vi "STED Control V3.vi"() -> ()   [LabVIEW 2014]
uses:
  FPGA-7842R-Reference.ctl
  Scan Parameters.ctl
  Manual Controls V2.ctl
  <vilib>/Utility/miscctls.llb/LVRectTypeDef.ctl
  <vilib>/Utility/miscctls.llb/LVPositionTypeDef.ctl
  Laser Controls.ctl
  XY_Stage/StageStates.ctl
  Type Defs/Image Acquisition Parameters.ctl
  Detectors.ctl
  Stage Control.ctl
panel:
  in  "Manual Controls":T1={"Galvo 1 Position (I16)"=-280, "Galvo 2 Position (I16)"=0, "X Axis Voltage (I16)"=0, "Y Axis Voltage (I16)"=0, "Z Axis Voltage (I16)"=0, "Res Mirror Amp (I16)"=0, "Res Mirror Mute"=FALSE}
  in  "Stage Control":T2={"Halt"=FALSE, "Home"=FALSE, "Down Stage"=FALSE, "Right Stage"=FALSE, "Up Stage"=FALSE, "Left Stage"=FALSE, "Mode"=enum."Joystick", "X Position"=1.0, "Y Position"=1.0, "Step Size (um)"=enum."1", "Velocity"=enum."Low"} {"Y Position" min=1.0 max=24.0; "X Position" min=1.0 max=24.0}
  in  "Move XY Stage":bool
  in  "Autoscale Z":bool
  in  "Reset Zoom":bool
  in  "Zoom Out":bool
  in  "Zoom In":bool
  in  "Pan":bool
  in  "Remove Display":bool
  in  "Add Display":bool
  in  "Colormap 2":u16(ring) items=["Fire", "Gray", "Red", "Green", "Blue", "Cyan", "Magenta", "Yellow", "Red-White", "Green-White", "Blue-White", "Glow"]
  in  "Merge Tool":bool
  in  "Smooth Tool":bool
  out "Channel 6":sgl[][](graph)
  out "Channel 5":sgl[][](graph)
  out "Channel 4":sgl[][](graph)
  out "Channel 3":sgl[][](graph)
  out "Channel 2":sgl[][](graph)
  in  "Dual Screens":bool=TRUE
  in  "Detectors":T3
  in  "Laser Controls":T4 {"590 Power (V)" scale=0.0..3.0; "STED Power (V)" scale=0.0..5.0}
  in  "Save File Path":path
  in  "Capture":bool
  in  "show cursor":bool
  in  "Set Mode Offset":bool
  in  "Unused Axis Voltage":i16=16300
  out "Channel 1":sgl[][](graph)
  in  "Image Acquisition Parameters":T5={"Scan Type"=enum."Sample Scanning", "Scan Mode"=enum."XY", "Fast Axis Frequency (Hz)"=100.0, "Image Format"=128, "Line Accumulations"=1, "Frames Per Capture"=1, "Frames Accumulations"=1, "Image Dimension (um)"=[], "Number of Z Steps"=1, "Z Steps Size (um)"=1.0, "Pixel Size (nm)"=[]} {"Z Steps Size (um)" min=0.0; "Number of Z Steps" min=1; "Frames Accumulations" min=1; "Frames Per Capture" min=1; "Line Accumulations" min=1; "Image Format" items=["64 x 64"=64, "128 x 128"=128, "256 x 256"=256, "512 x 512"=512, "1024 x 1024"=1024, "2048 x 2048"=2048]}
  in  "Live":bool
  in  "Exit":bool
  # "XY"
  # "Z"
  # "Length"
  # "Height"
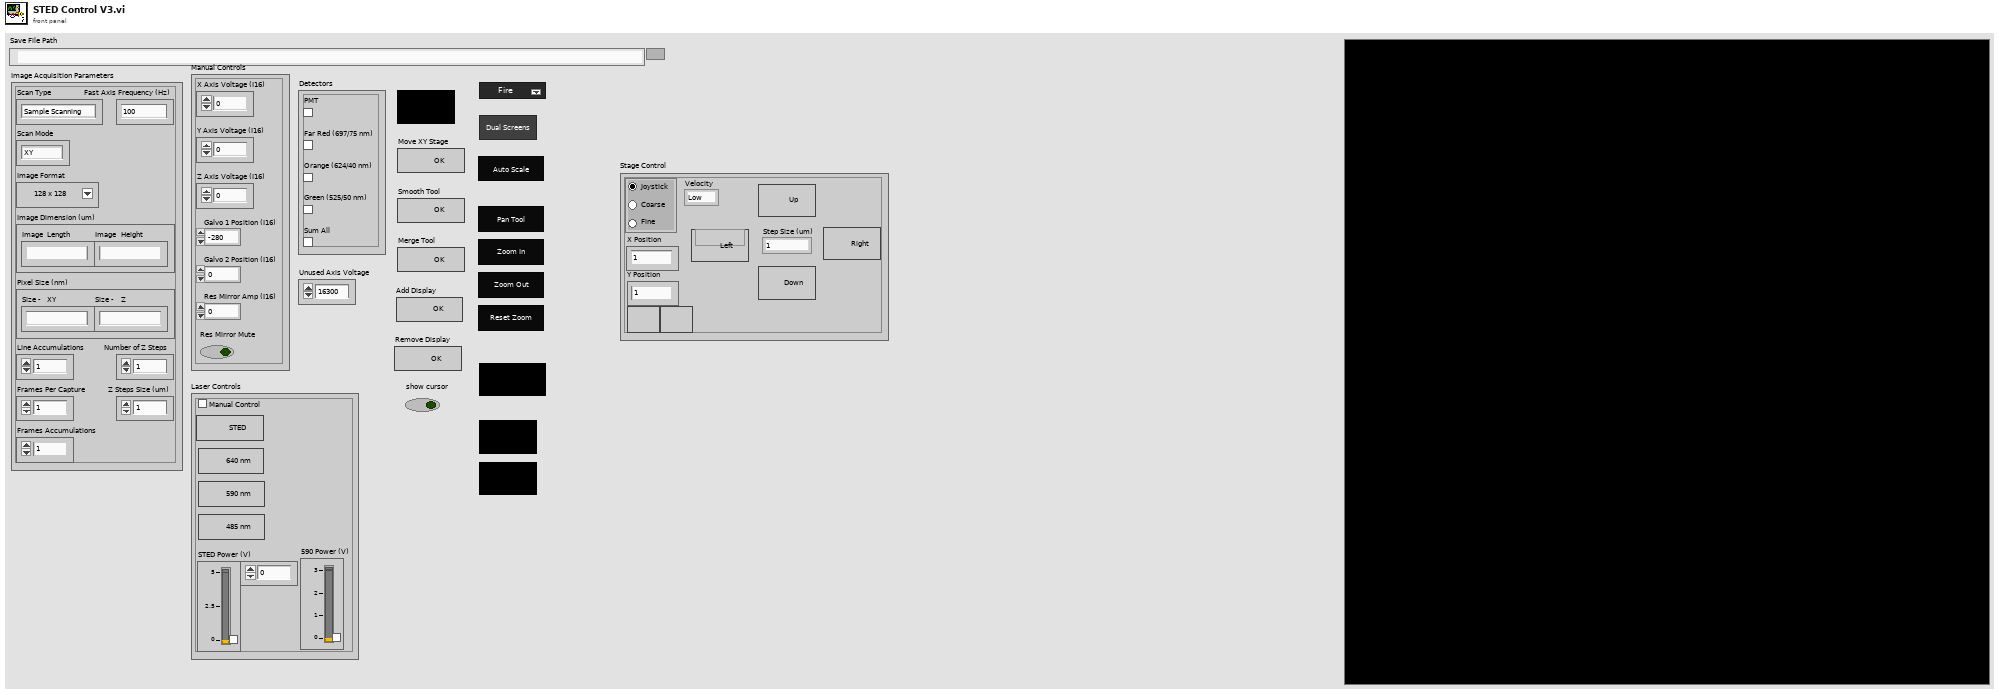
[diagram p1: front panel]
types:
  T1 = typedef "Manual Controls V2.ctl" = cluster{"Galvo 1 Position (I16)":i16, "Galvo 2 Position (I16)":i16, "X Axis Voltage (I16)":i16, "Y Axis Voltage (I16)":i16, "Z Axis Voltage (I16)":i16, "Res Mirror Amp (I16)":i16, "Res Mirror Mute":bool}
  T2 = typedef "Stage Control.ctl" = cluster{"Halt":bool, "Home":bool, "Down Stage":bool, "Right Stage":bool, "Up Stage":bool, "Left Stage":bool, "Mode":enum32{"Joystick", "Coarse", "Fine"}, "X Position":dbl, "Y Position":dbl, "Step Size (um)":enum16{"1", "2", "5", "10", "15", "20", "50", "100", "500"}, "Velocity":enum16{"Low", "Medium", "High"}}
  T3 = typedef "Detectors.ctl" = cluster{"PMT":bool, "Far Red (697/75 nm)":bool, "Orange (624/40 nm)":bool, "Green (525/50 nm)":bool, "Sum All":bool}
  T4 = typedef "Laser Controls.ctl" = cluster{"STED Power (V)":dbl, "590 Power (V)":dbl, "STED":bool, "640 nm":bool, "590 nm":bool, "485 nm":bool, "Manual Control":bool}
  T5 = typedef "Image Acquisition Parameters.ctl" = cluster{"Scan Type":enum16{"Sample Scanning", "Beam Scanning"}, "Scan Mode":enum16{"XY", "XZ", "YZ", "XYZ"}, "Fast Axis Frequency (Hz)":dbl, "Image Format":u16, "Line Accumulations":u16, "Frames Per Capture":u16, "Frames Accumulations":u16, "Image Dimension (um)":dbl[], "Number of Z Steps":u8, "Z Steps Size (um)":dbl, "Pixel Size (nm)":dbl[]}
  T6 = typedef "Scan Parameters.ctl" = cluster{"Fast_Ax_Amp_V":dbl, "Fast_Ax_Off_V":dbl, "Slow_Ax_Amp_V":dbl, "Slow_Ax_Off_V ":dbl, "Slow_Ax_Max_V_VperS":dbl, "Slow_Ax1_Del25ns":i32, "Slow_Ax2_Del25ns":i32, "Stage_X_Off_V":dbl, "Stage_Y_Off_V":dbl, "Stage_Z_Off_V":dbl, "Galvo1_Off_V":dbl, "Galvo2_Off_V":dbl, "Last_Scan_Mode":enum16{"XY", "XZ", "YZ", "XYZ"}, "Current_Scan_Mode":enum16{"XY", "XZ", "YZ", "XYZ"}, "Fly_Back_Lines":u16, "Linear_Ramp_End":u32, "Z_Step_I16":i16, "Z_Start_I16":i16, "Laser_States _U32":u32, "590_Voltage_I16":i16, "775_AOM_Volt_I16":i16, "Blanking OFF":bool, "Unused_Axis_I16":i16}
  T7 = typedef "FPGA-7842R-Reference.ctl" = enum16{"Stage Control", "Laser Control", "Unused Axis I16", "Exit", "Set Res Mirror", "Set Galvo", "Default", "Close FPGA", "Stop Waveforms", "Start Waveforms", "Initialize"}
  T8 = typedef "LVPositionTypeDef.ctl" = cluster{"Left":i32, "Top":i32}
  T9 = typedef "LVRectTypeDef.ctl" = cluster{"Left":i16, "Top":i16, "Right":i16, "Bottom":i16}
  T10 = enum32{"Invalid", "Standard", "Closed", "Hidden", "Minimized", "Maximized"}
  T11 = typedef "StageStates.ctl" = enum16{"POSITION", "MVR", "MOVE", "HALT", "ONTARGET", "ERROR", "EXIT", "HOME", "ZEROPOS", "NANOPOS", "QUIT", "SERVO", "JOYSTICK", "ANALOG"}
  T12 = typedef "LVRangeTypeDef.ctl" = cluster{"Minimum":dbl, "Maximum":dbl, "Increment":dbl, "Minor Increment":dbl, "Start":dbl}
  T13 = typedef "LVAllMonitorsDisplayTypeDef.ctl" = cluster{"Bounds":cluster{"Left":i16, "Top":i16, "Right":i16, "Bottom":i16}, "Depth":i16}[]
  T14 = cluster{"Bounds":cluster{"Left":i16, "Top":i16, "Right":i16, "Bottom":i16}, "Depth":i16}
  T15 = cluster{"Halt":bool, "Home":bool, "Down Stage":bool, "Right Stage":bool, "Up Stage":bool, "Left Stage":bool, "Mode":bool, "X Position":bool, "Y Position":bool, "Step Size (um)":bool, "Velocity":bool}
  T16 = enum16{"1", "2", "5", "10", "15", "20", "50", "100", "500"}
  T17 = typedef "Scanning Conversions.ctl" = cluster{"Stage X Axis (Volts/um)":dbl, "Stage Y Axis (Volts/um)":dbl, "Stage Z Axis (Volts/um)":dbl}
  T18 = typedef "IMAQ Image.ctl" = refnum<image>
  T19 = typedef "Waveform Data.ctl" = cluster{"Waveform Scan Parameters":cluster{"Scanning Mode":u8, "Fast Axis WF Length (Elements)":i32, "Fast Axis Sample Period (Ticks)":u32, "Slow Axis 1 WF Length (Elements)":i32, "Slow Axis 1 Sample Period (Ticks)":u32, "Slow Axis 1 Delay (25 ns) Steps":i32, "Slow Axis 2 WFLength (Elements)":i32, "Slow Axis 2 Sample Period (Ticks)":u32, "Slow Axis 2 Delay (25 ns) Steps":i32}, "Fast Axis Waveform":dbl[], "Slow Axis 1 Waveform":dbl[], "Slow Axis 2 Waveform":dbl[]}
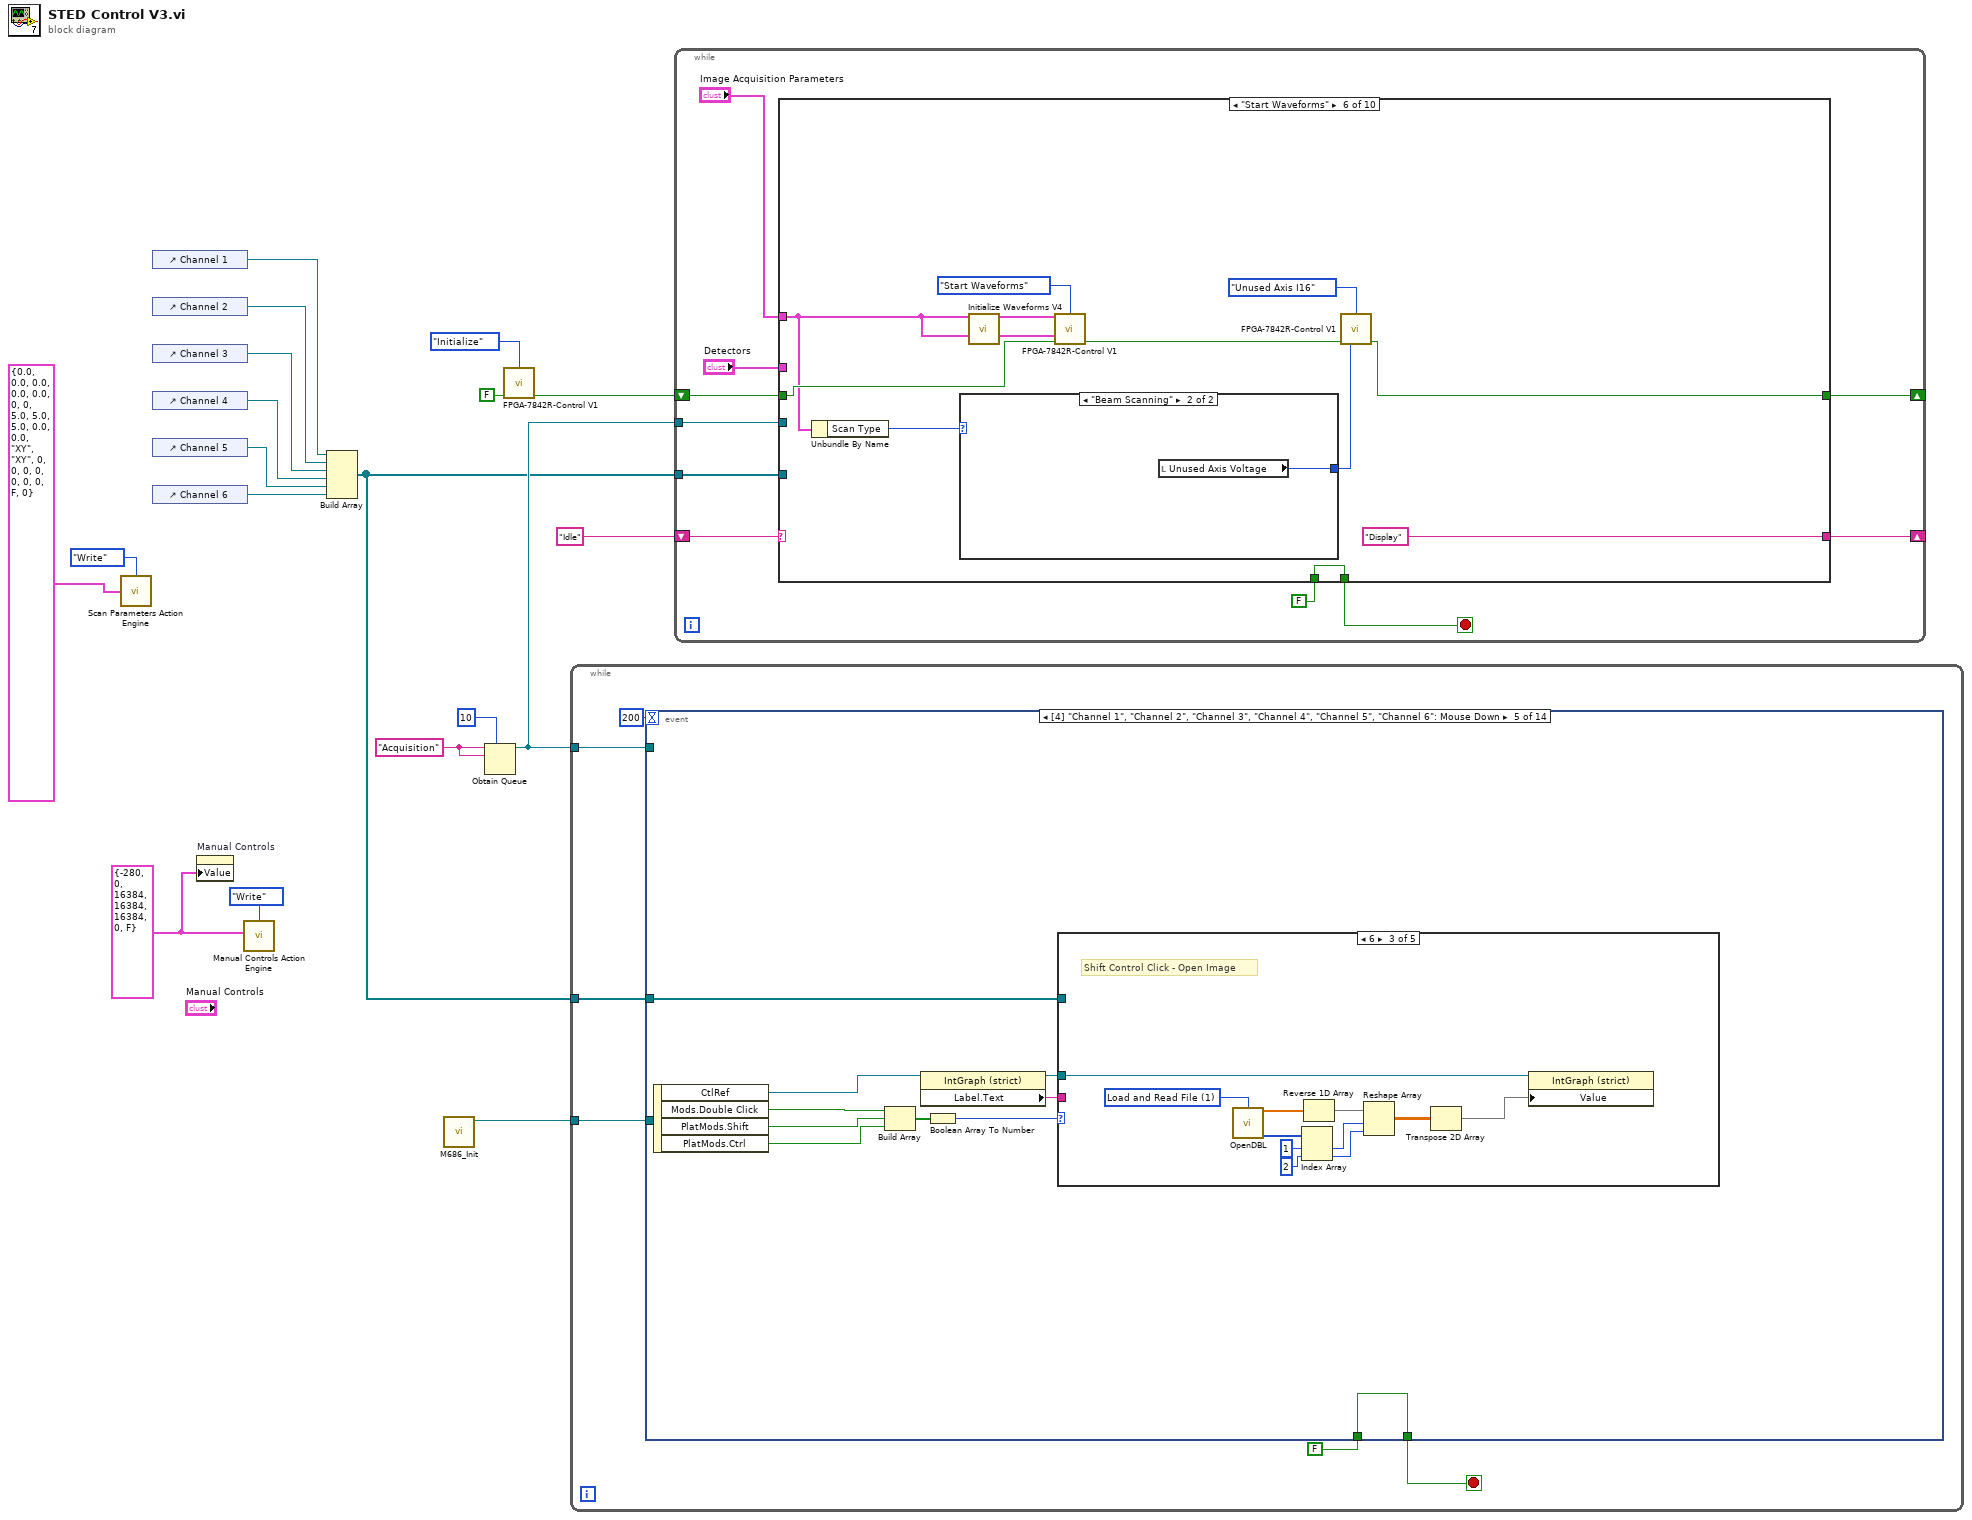
[diagram p0: block diagram]
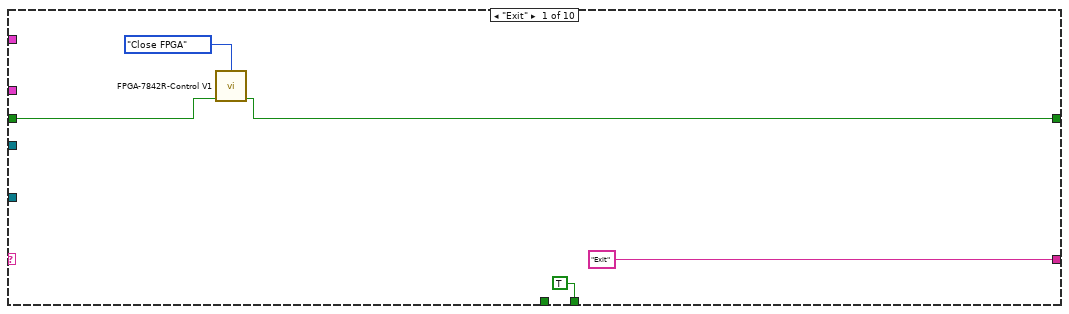
[diagram p2: hidden frame]
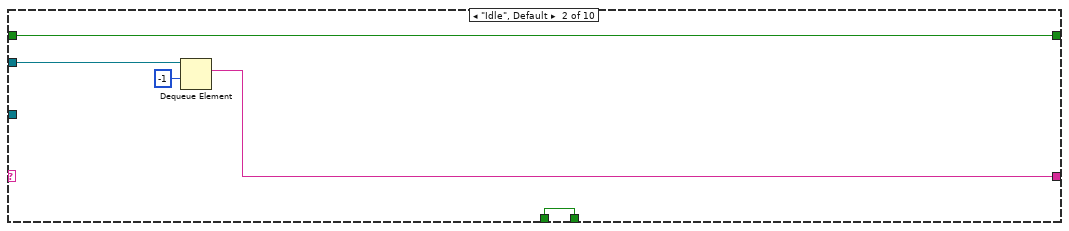
[diagram p3: hidden frame]
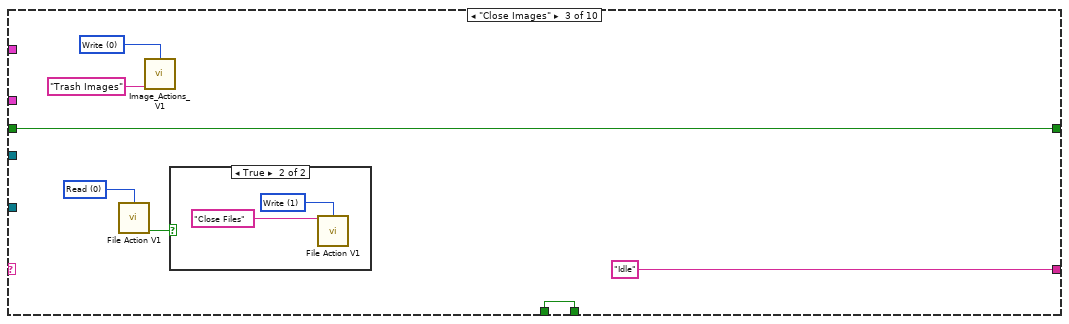
[diagram p4: hidden frame]
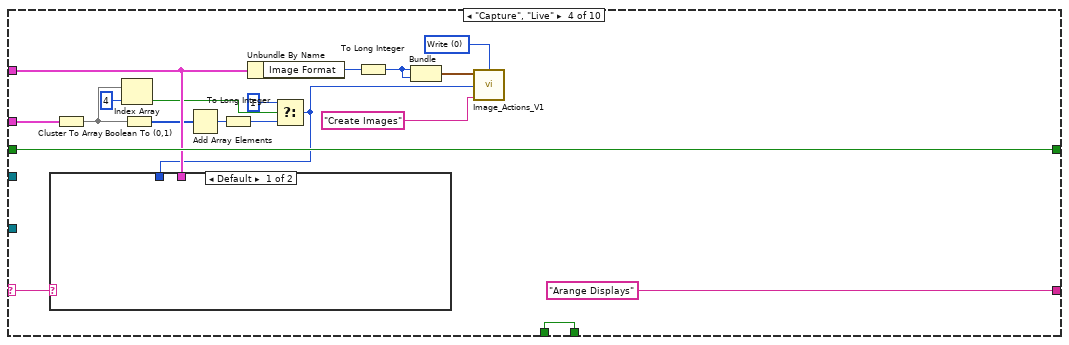
[diagram p6: hidden frame]
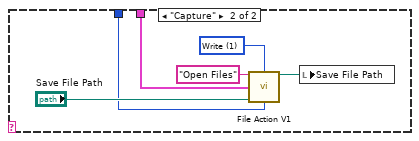
[diagram p7: hidden frame]
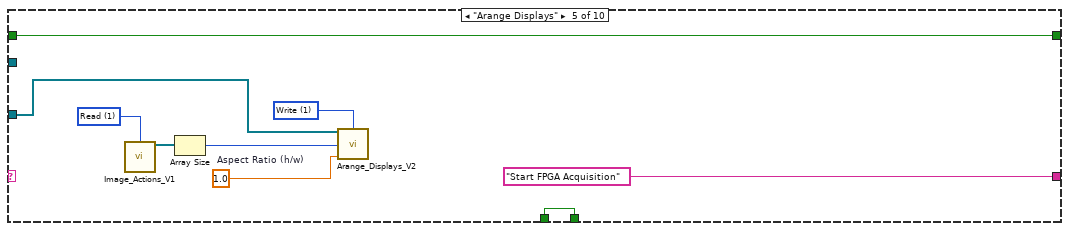
[diagram p8: hidden frame]
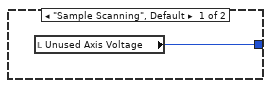
[diagram p9: hidden frame]
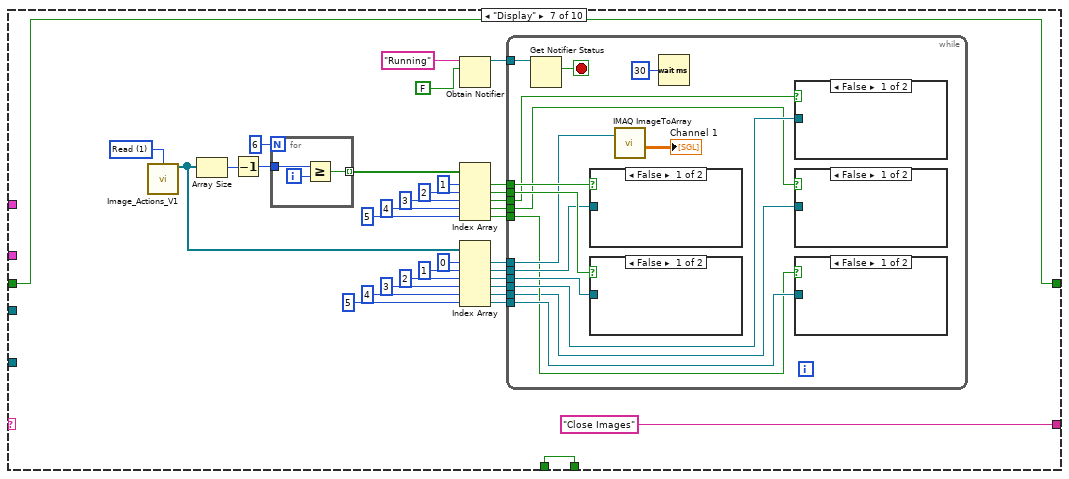
[diagram p10: hidden frame]
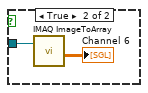
[diagram p11: hidden frame]
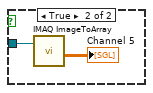
[diagram p12: hidden frame]
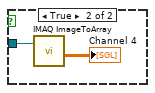
[diagram p13: hidden frame]
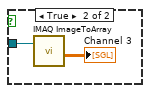
[diagram p14: hidden frame]
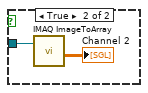
[diagram p15: hidden frame]
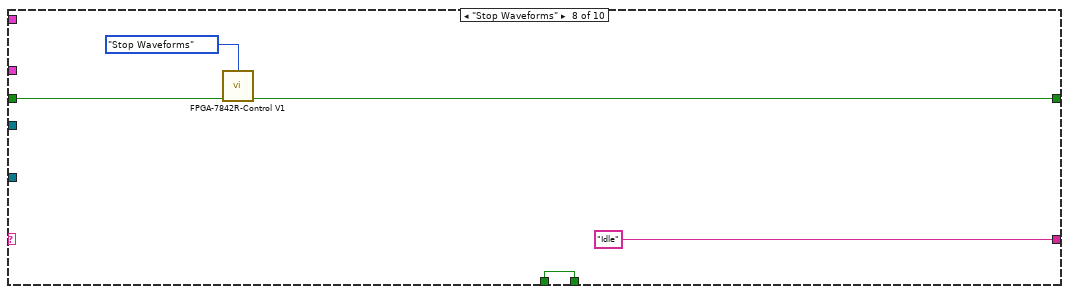
[diagram p16: hidden frame]
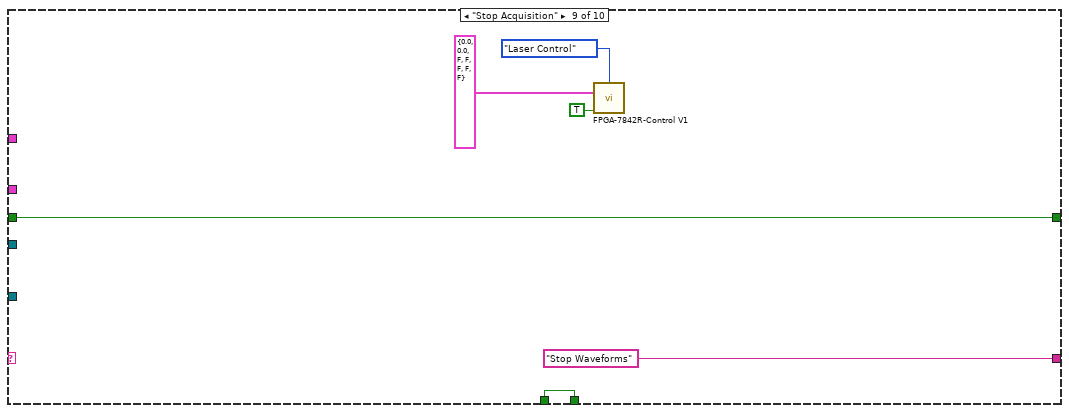
[diagram p17: hidden frame]
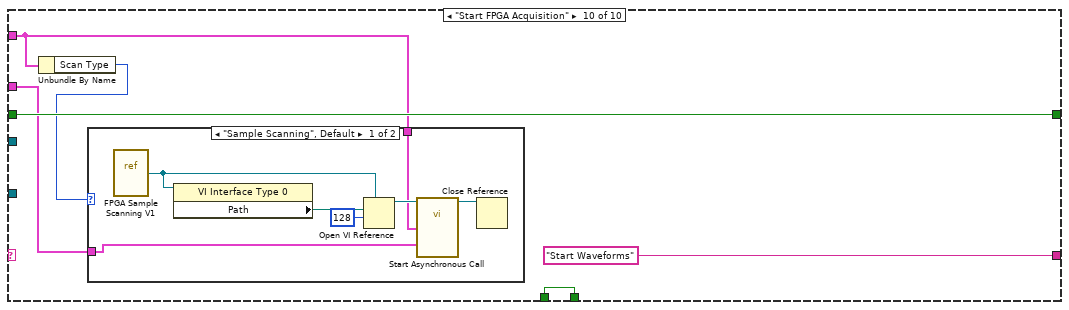
[diagram p18: hidden frame]
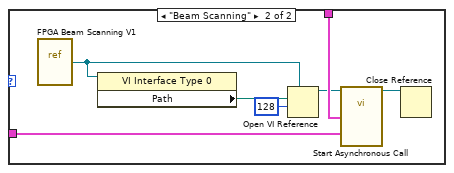
[diagram p19: hidden frame]
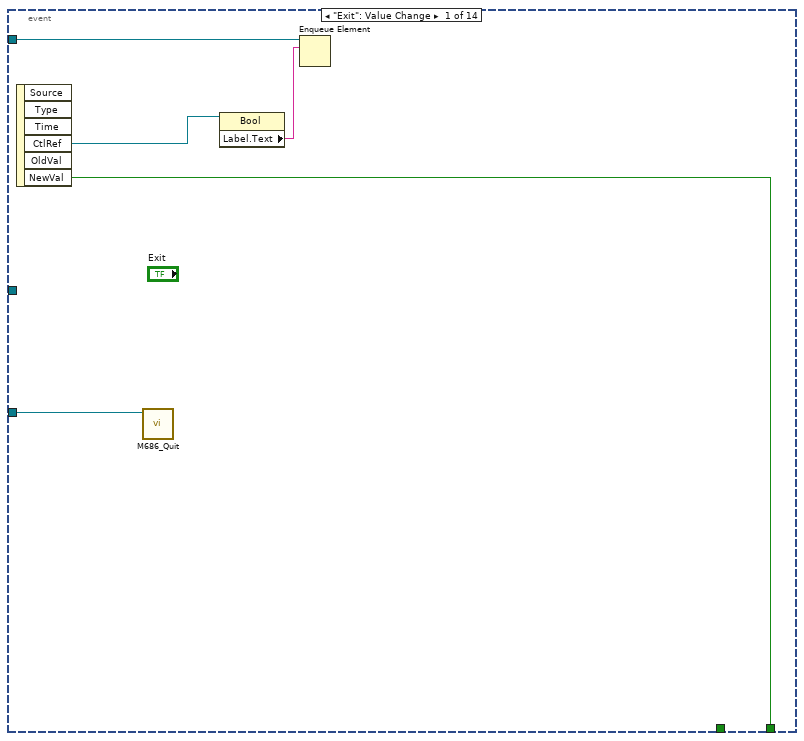
[diagram p20: hidden frame]
diagram:
  w1 = T1 {"Galvo 1 Position (I16)"=-280, "Galvo 2 Position (I16)"=0, "X Axis Voltage (I16)"=16384, "Y Axis Voltage (I16)"=16384, "Z Axis Voltage (I16)"=16384, "Res Mirror Amp (I16)"=0, "Res Mirror Mute"=FALSE} ("Manual Controls")
  w18 = "Acquisition" ("name (unnamed)")
  n1 = call "Scan Parameters Action Engine.vi"("Action"=enum16{"Read", "Write"}."Write", "Scan Parameters IN"=T6 {"Fast_Ax_Amp_V"=0.0, "Fast_Ax_Off_V"=0.0, "Slow_Ax_Amp_V"=0.0, "Slow_Ax_Off_V "=0.0, "Slow_Ax_Max_V_VperS"=0.0, "Slow_Ax1_Del25ns"=0, "Slow_Ax2_Del25ns"=0, "Stage_X_Off_V"=5.0, "Stage_Y_Off_V"=5.0, "Stage_Z_Off_V"=5.0, "Galvo1_Off_V"=0.0, "Galvo2_Off_V"=0.0, "Last_Scan_Mode"=enum."XY", "Current_Scan_Mode"=enum."XY", "Fly_Back_Lines"=0, "Linear_Ramp_End"=0, "Z_Step_I16"=0, "Z_Start_I16"=0, "Laser_States _U32"=0, "590_Voltage_I16"=0, "775_AOM_Volt_I16"=0, "Blanking OFF"=FALSE, "Unused_Axis_I16"=0}) -> ()  [unwired: 13 in, 1 out]
  n2 = control-ref of="Channel 1"() -> (w10:refnum<vi>)
  n3 = control-ref of="Channel 2"() -> (w9:refnum<vi>)
  n4 = control-ref of="Channel 3"() -> (w8:refnum<vi>)
  n5 = control-ref of="Channel 4"() -> (w7:refnum<vi>)
  n6 = control-ref of="Channel 5"() -> (w6:refnum<vi>)
  n7 = control-ref of="Channel 6"() -> (w5:refnum<vi>)
  n8 = property on="Manual Controls" class="Clust (strict)"("Value"=w1) -> ()  [unwired: 2 in, 2 out]
  n9 = call "Manual Controls Action Engine.vi"("Action"=enum16{"Read", "Write"}."Write", "Manual Controls In"=w1) -> ()  [unwired: 13 in, 1 out]
  n10 = Build Array(w10, w9, w8, w7, w6, w5) -> (w4:refnum<vi>[])
  n11 = call "M686_Init.vi"() -> ("VISA Refnum out"=w2:refnum<visa-resource-name>)  [unwired: 9 in, 2 out]
  n12 = Obtain Queue(max queue size (-1, unlimited)=10, name (unnamed)=w18, element data type=w18) -> (queue out=w16:refnum<queue>)  [unwired: 2 in, 2 out]
  n13 = call "FPGA-7842R-Control V1.vi"("Action"=FPGA-7842R-Reference."Initialize", "Initialize"=FALSE) -> ("Initalized"=w13:bool)  [unwired: 13 in]
  n14 = while {
    tunnel: w16 -> [w23]
    tunnel: w4 -> [w21]
    tunnel: w2 -> [w20]
    stop <- w25 stop-if-true
    n15 = event shown="[4] \"Channel 1\", \"Channel 2\", \"Channel 3\", \"Channel 4\", \"Channel 5\", \"Channel 6\": Mouse Down" {
      selector: _ -> [_ _ _ _ _ _ _ _ _ _ _ _ _ _]
      dyn-events: _ -> [_ _ _ _ _ _ _ _ _ _ _ _ _ _]
      timeout: 200 -> [_ _ _ _ _ _ _ _ _ _ _ _ _ _]
      tunnel: [w30 w42 w47 w85 w112 w177 w197 w205 w232 w285 w414 w415 w595 w807] -> w25
      tunnel: FALSE -> [_ w42 w47 w85 w112 w177 w197 w205 w232 w285 w414 w415 w595 w807]
      tunnel: w23 -> [w29 w41 _ _ _ _ w191 _ _ _ _ _ _ _]
      tunnel: w21 -> [_ _ w44 _ w107 w176 _ _ _ _ _ _ _ _]
      tunnel: w20 -> [w26 _ _ _ _ _ _ _ _ _ _ w424 _ _]
      event "Exit": Value Change {
        n16 = event-data() -> ("CtlRef"=w28:refnum<vi>, "NewVal"=w30:bool)  [unwired: 1 in, 4 out]
        n17 = call "M686_Quit.vi"("VISA Refnum in"=w26) -> ()  [unwired: 11 in]
        n18 = property class="Bool"(reference=w28) -> ("Label.Text"=w27:string)  [unwired: 1 in, 2 out]
        n19 = Enqueue Element(queue=w29, element=w27) -> ()  [unwired: 2 in, 3 out]
      }
      event "Live", "Capture": Value Change {
        n20 = event-data() -> ("CtlRef"=w40:refnum<vi>, "NewVal"=w32:bool)  [unwired: 1 in]
        n21 = property on="Channel 1" class="IntGraph (strict)"("Cursor.Visible"=FALSE) -> ()  [unwired: 2 in, 2 out]
        n22 = property class="Bool (strict)"(reference=w40) -> ("Label.Text"=w31:string)  [unwired: 1 in, 2 out]
        n23 = Obtain Notifier(name (unnamed)="Running", notification data type=TRUE) -> (notifier out=w37:refnum<notifier>)  [unwired: 2 in, 2 out]
        n24 = Not(x=w32) -> (.not. x?=w35:bool)
        n25 = Send Notification(notification=w35, notifier=w37) -> ()  [unwired: 1 in, 2 out]
        n26 = Select(t=w31, s=w32, f="Stop Acquisition") -> (s? t:f=w33:string)
        n27 = Enqueue Element(queue=w41, element=w33) -> ()  [unwired: 2 in, 3 out]
      }
      event "Smooth Tool", "Merge Tool", "Add Display", "Remove Display", "Autoscale Z", "Move XY Stage": Value Change {
        n28 = event-data() -> ("CtlRef"=w46:refnum<vi>)  [unwired: 1 in, 5 out]
        n29 = property class="Bool"(reference=w46) -> ("Label.Text"=w45:string)  [unwired: 1 in, 2 out]
        n30 = control-ref of="This VI"() -> (w43:refnum<vi>)
        n31 = case shown="\"Autoscale Z\"" w45 {
          tunnel: w44 -> [_ w49 w56 _ w66 w70 w76]
          tunnel: w43 -> [_ w48 _ _ _ _ w75]
          frame Default {
          }
          frame "Merge Tool" {
            n32 = vi-ref "MergeTool - Cambridge.vi"() -> (w53:refnum<vi>)
            n33 = property class="VI Interface Type 2"(reference=w53) -> ("Path"=w51:path)  [unwired: 1 in, 2 out]
            n34 = Open VI Reference(type specifier VI Refnum (for type only)=w53, vi path=w51, options=128) -> (vi reference=w52:refnum<vi>)  [unwired: 3 in, 1 out]
            n35 = call-by-ref "Start Asynchronous Call"(reference=w52, "VI Reference"=w48, "Display References"=w49) -> (reference out=w54:refnum<vi>)  [unwired: 11 in, 1 out]
            n36 = Close Reference(reference=w54) -> ()  [unwired: 1 in, 1 out]
          }
          frame "Add Display" {
            w59 = u16 1 items=["Read", "Write"] ("Action")
            w60 = u16 0 items=["Read", "Write"] ("Action")
            n37 = call "Arange_Displays_V2.vi"("Action"=w60) -> ("Number of Channels OUT"=w58:i32)  [unwired: 14 in]
            n38 = Increment(x=w58) -> (x+1=w57:i32)
            n39 = call "Arange_Displays_V2.vi"("Display References"=w56, "Action"=w59, "Number of Channels"=w57, "Aspect Ratio (h/w)"=1.0) -> ()  [unwired: 11 in, 1 out]
          }
          frame "Move XY Stage" {
            n40 = vi-ref "StageController_V2.vi"() -> (w64:refnum<vi>)
            n41 = property class="VI Interface Type 3"(reference=w64) -> ("Path"=w62:path)  [unwired: 1 in, 2 out]
            n42 = Open VI Reference(type specifier VI Refnum (for type only)=w64, vi path=w62, options=128) -> (vi reference=w63:refnum<vi>)  [unwired: 3 in, 1 out]
            n43 = call-by-ref "Start Asynchronous Call"(reference=w63) -> (reference out=w65:refnum<vi>)  [unwired: 13 in, 1 out]
            n44 = Close Reference(reference=w65) -> ()  [unwired: 1 in, 1 out]
          }
          frame "Autoscale Z" {
            n45 = for {
              tunnel: w66 -> [w67] mode=indexing
              n46 = property class="IntGraph (strict)"(reference=w67, "ZScale.ScaleFit"=u8 1 ("Z Scale.Scale Fit")) -> ()  [unwired: 1 in, 2 out]
            }
          }
          frame "Remove Display" {
            w73 = u16 1 items=["Read", "Write"] ("Action")
            w74 = u16 0 items=["Read", "Write"] ("Action")
            n47 = call "Arange_Displays_V2.vi"("Action"=w74) -> ("Number of Channels OUT"=w72:i32)  [unwired: 14 in]
            n48 = Decrement(x=w72) -> (x-1=w71:i32)
            n49 = call "Arange_Displays_V2.vi"("Display References"=w70, "Action"=w73, "Number of Channels"=w71, "Aspect Ratio (h/w)"=1.0) -> ()  [unwired: 11 in, 1 out]
          }
          frame "Smooth Tool" {
            n50 = vi-ref "SmoothTool.vi"() -> (w78:refnum<vi>)
            n51 = property class="VI Interface Type 3"(reference=w78) -> ("Path"=w80:path)  [unwired: 1 in, 2 out]
            n52 = Open VI Reference(type specifier VI Refnum (for type only)=w78, vi path=w80, options=128) -> (vi reference=w79:refnum<vi>)  [unwired: 3 in, 1 out]
            n53 = call-by-ref "Start Asynchronous Call"(reference=w79, "VI Reference"=w75, "Display References"=w76) -> (reference out=w77:refnum<vi>)  [unwired: 2 in, 1 out]
            n54 = Close Reference(reference=w77) -> ()  [unwired: 1 in, 1 out]
          }
        }
      }
      event "Pan", "Zoom In", "Zoom Out", "Reset Zoom": Value Change {
        n55 = event-data() -> ("CtlRef"=w83:refnum<vi>, "NewVal"=w82:bool)  [unwired: 1 in]
        n56 = case shown="True" w82 {
          tunnel: w83 -> [_ w93]
          tunnel: [0 ("Palette:Active Tool") w92] -> w84
          frame False {
          }
          frame True {
            n57 = property class="Bool (strict)"(reference=w93) -> ("Label.Text"=w87:string)  [unwired: 1 in, 2 out]
            n58 = Build Array("Pan", "Zoom In", "Zoom Out") -> (w88:string[])
            n59 = case shown="\"Pan\"" w87 {
              tunnel: [6 ("Palette:Active Tool") 7 ("Palette:Active Tool") 5 ("Palette:Active Tool") 1 ("Palette:Active Tool")] -> w92
              frame "Zoom In" {
              }
              frame "Zoom Out" {
              }
              frame "Reset Zoom", Default {
              }
              frame "Pan" {
              }
            }
            n60 = for {
              tunnel: w88 -> [w94] mode=indexing
              tunnel: w87 -> [w98]
              n61 = Equal?(x=w98, y=w94) -> (x = y?=w95:bool)
              n62 = control-ref of="This VI"() -> (w96:refnum<vi>)
              n63 = To Variant(anything=w95) -> (Variant=w97:variant)
              n64 = invoke class="VI" method="Ctrl Val.Set"(reference=w96, "Control Name"=w94, "Value"=w97) -> ()  [unwired: 2 in, 5 out]
            }
          }
        }
        n65 = property on="Channel 1" class="IntGraph (strict)"("ActPaletteTool"=w84) -> ()  [unwired: 2 in, 2 out]
        n66 = property on="Channel 2" class="IntGraph (strict)"("ActPaletteTool"=w84) -> ()  [unwired: 2 in, 2 out]
        n67 = property on="Channel 3" class="IntGraph (strict)"("ActPaletteTool"=w84) -> ()  [unwired: 2 in, 2 out]
        n68 = property on="Channel 4" class="IntGraph (strict)"("ActPaletteTool"=w84) -> ()  [unwired: 2 in, 2 out]
        n69 = property on="Channel 5" class="IntGraph (strict)"("ActPaletteTool"=w84) -> ()  [unwired: 2 in, 2 out]
        n70 = property on="Channel 6" class="IntGraph (strict)"("ActPaletteTool"=w84) -> ()  [unwired: 2 in, 2 out]
      }
      event "Channel 1", "Channel 2", "Channel 3", "Channel 4", "Channel 5", "Channel 6": Mouse Down {
        n71 = event-data() -> ("CtlRef"=w108:refnum<vi>, "Mods.Double Click"=w111:bool, "PlatMods.Shift"=w110:bool, "PlatMods.Ctrl"=w109:bool)  [unwired: 1 in]
        n72 = Build Array(w111, w110, w109) -> (w104:bool[])
        n73 = property class="IntGraph (strict)"(reference=w108) -> (reference out=w106:refnum<vi>, "Label.Text"=w103:string)  [unwired: 1 in, 1 out]
        n74 = Boolean Array To Number(Boolean array=w104) -> (number=w105:u32)
        n75 = case shown="6" w105 {
          tunnel: w103 -> [w114 _ _ _ _]
          tunnel: w106 -> [_ w129 w164 w175 _]
          tunnel: w107 -> [w113 _ _ _ _]
          frame 0 {
            n76 = for {
              tunnel: w114 -> [w118]
              tunnel: w113 -> [w117] mode=indexing
              # "Single Click - Show Z Scale"
              n77 = property class="IntGraph (strict)"(reference=w117) -> (reference out=w115:refnum<vi>, "Label.Text"=w116:string)  [unwired: 1 in, 1 out]
              n78 = Equal?(x=w116, y=w118) -> (x = y?=w120:bool)
              n79 = Select(t=T8 {"Left"=2000, "Top"=17} ("Z Scale.Position"), s=w120, f=T8 {"Left"=0, "Top"=0} ("Z Scale.Position")) -> (s? t:f=w119:T8)
              n80 = property class="IntGraph (strict)"(reference=w115, "ZScale.Visible"=w120, "ZScale.Position"=w119) -> ()  [unwired: 1 in, 2 out]
            }
          }
          frame 2 {
            # "Shift Click - Apply color map."
            n81 = property class="IntGraph (strict)"(reference=w129) -> (reference out=w123:refnum<vi>, "ZScale.Maximum"=w124:dbl)  [unwired: 1 in, 1 out]
            n82 = case shown="0, Default" "Colormap 2" {
              tunnel: [cluster{dbl, u32}[] [{0.0, 0}, {85.0, 16711680}, {108.0, 16729344}, {127.0, 16744192}, {132.0, 16747520}, {140.0, 16753920}, {157.0, 16766720}, {170.0, 16776960}, {245.0, 16777184}, {250.0, 16777200}, {255.0, 16777215}] ("Z Scale.Marker Values[]") cluster{dbl, u32}[] [{0.0, 0}, {255.0, 16777215}] ("Z Scale.Marker Values[]") cluster{dbl, u32}[] [{0.0, 0}, {255.0, 16711680}] ("Z Scale.Marker Values[]") cluster{dbl, u32}[] [{0.0, 0}, {255.0, 65280}] ("Z Scale.Marker Values[]") cluster{dbl, u32}[] [{0.0, 0}, {255.0, 255}] ("Z Scale.Marker Values[]") cluster{dbl, u32}[] [{0.0, 0}, {255.0, 65535}] ("Z Scale.Marker Values[]") cluster{dbl, u32}[] [{0.0, 0}, {255.0, 16711935}] ("Z Scale.Marker Values[]") cluster{dbl, u32}[] [{0.0, 0}, {255.0, 16776960}] ("Z Scale.Marker Values[]") cluster{dbl, u32}[] [{0.0, 0}, {170.0, 16711680}, {245.0, 16777184}, {250.0, 16777200}, {255.0, 16448250}] ("Z Scale.Marker Values[]") cluster{dbl, u32}[] [{0.0, 0}, {170.0, 65280}, {245.0, 16777184}, {250.0, 16777200}, {255.0, 16448250}] ("Z Scale.Marker Values[]") cluster{dbl, u32}[] [{0.0, 0}, {170.0, 255}, {245.0, 16777184}, {250.0, 16777200}, {255.0, 16448250}] ("Z Scale.Marker Values[]") cluster{dbl, u32}[] [{0.0, 0}, {1.0, 131072}, {2.0, 196608}, {3.0, 327680}, {4.0, 458752}, {5.0, 589824}, {6.0, 720896}, {7.0, 851971}, {8.0, 983043}, {9.0, 1114115}, {10.0, 1245187}, {11.0, 1376259}, {12.0, 1507331}, {13.0, 1638403}, {14.0, 1769475}, {15.0, 1769479}, {16.0, 2031623}, {17.0, 2162695}, {18.0, 2293767}, {19.0, 2424839}, {20.0, 2555911}, {21.0, 2686983}, {22.0, 2818055}, {23.0, 2949127}, {24.0, 3080203}, {25.0, 3211275}, {26.0, 3342347}, {27.0, 3473419}, {28.0, 3604491}, {29.0, 3735563}, {30.0, 3866635}, {31.0, 3867403}, {32.0, 4129547}, {33.0, 4260619}, {34.0, 4391691}, {35.0, 4522763}, {36.0, 4653839}, {37.0, 4784911}, {38.0, 4915983}, {39.0, 5178127}, {40.0, 5309199}, {41.0, 5440271}, {42.0, 5571343}, {43.0, 5702415}, {44.0, 5703439}, {45.0, 5965583}, {46.0, 6096655}, {47.0, 6227727}, {48.0, 6358799}, {49.0, 6489871}, {50.0, 6620943}, {51.0, 6752015}, {52.0, 6883087}, {53.0, 7015183}, {54.0, 7146255}, {55.0, 7277327}, {56.0, 7408399}, {57.0, 7539471}, {58.0, 7670543}, {59.0, 7801615}, {60.0, 8063759}, {61.0, 8194831}, {62.0, 8326927}, {63.0, 8457999}, {64.0, 8589075}, {65.0, 8720147}, {66.0, 8851219}, {67.0, 8982291}, {68.0, 9113363}, {69.0, 9114387}, {70.0, 9376531}, {71.0, 9507603}, {72.0, 9638675}, {73.0, 9769747}, {74.0, 9901843}, {75.0, 10032915}, {76.0, 10163987}, {77.0, 10229523}, {78.0, 10295059}, {79.0, 10427155}, {80.0, 10558227}, {81.0, 10689299}, {82.0, 10820371}, {83.0, 10886931}, {84.0, 10952467}, {85.0, 11083539}, {86.0, 11214611}, {87.0, 11215635}, {88.0, 11477779}, {89.0, 11543315}, {90.0, 11608851}, {91.0, 11740947}, {92.0, 11806483}, {93.0, 11872019}, {94.0, 12004115}, {95.0, 12135187}, {96.0, 12266259}, {97.0, 12267283}, {98.0, 12398355}, {99.0, 12529427}, {100.0, 12530451}, {101.0, 12595987}, {102.0, 12530451}, {103.0, 12793619}, {104.0, 12794131}, {105.0, 12794643}, {106.0, 13056787}, {107.0, 13057299}, {108.0, 13057811}, {109.0, 13188883}, {110.0, 13320979}, {111.0, 13386515}, {112.0, 13452563}, {113.0, 13584147}, {114.0, 13584659}, {115.0, 13585171}, {116.0, 13585683}, {117.0, 13717267}, {118.0, 13848339}, {119.0, 13849363}, {120.0, 13849875}, {121.0, 13850387}, {122.0, 13981459}, {123.0, 14113555}, {124.0, 14114067}, {125.0, 14114579}, {126.0, 14115091}, {127.0, 14246675}, {128.0, 14377747}, {129.0, 14378771}, {130.0, 14379283}, {131.0, 14379539}, {132.0, 14379795}, {133.0, 14380819}, {134.0, 14511891}, {135.0, 14643987}, {136.0, 14644503}, {137.0, 14645015}, {138.0, 14645527}, {139.0, 14646039}, {140.0, 14646551}, {141.0, 14778135}, {142.0, 14909207}, {143.0, 14910231}, {144.0, 14910747}, {145.0, 14911259}, {146.0, 14911771}, {147.0, 14912283}, {148.0, 14912797}, {149.0, 15044383}, {150.0, 15175455}, {151.0, 15175967}, {152.0, 15176479}, {153.0, 15176991}, {154.0, 15177507}, {155.0, 15178019}, {156.0, 15178531}, {157.0, 15310115}, {158.0, 15441701}, {159.0, 15441959}, {160.0, 15442215}, {161.0, 15442727}, {162.0, 15443243}, {163.0, 15443755}, {164.0, 15444269}, {165.0, 15444783}, {166.0, 15444783}, {167.0, 15576367}, {168.0, 15707953}, {169.0, 15708467}, {170.0, 15708979}, {171.0, 15708981}, {172.0, 15708983}, {173.0, 15710011}, {174.0, 15710523}, {175.0, 15711037}, {176.0, 15711039}, {177.0, 15711553}, {178.0, 15843139}, {179.0, 15974213}, {180.0, 15974215}, {181.0, 15974217}, {182.0, 15974219}, {183.0, 15975755}, {184.0, 15976271}, {185.0, 15976785}, {186.0, 15977299}, {187.0, 15977301}, {188.0, 15977815}, {189.0, 15978327}, {190.0, 15978331}, {191.0, 16109917}, {192.0, 16241503}, {193.0, 16241505}, {194.0, 16242019}, {195.0, 16242535}, {196.0, 16242537}, {197.0, 16242539}, {198.0, 16243563}, {199.0, 16243567}, {200.0, 16244081}, {201.0, 16244595}, {202.0, 16244599}, {203.0, 16244601}, {204.0, 16244603}, {205.0, 16245627}, {206.0, 16245631}, {207.0, 16245633}, {208.0, 16246147}, {209.0, 16246663}, {210.0, 16377735}, {211.0, 16508811}, {212.0, 16508815}, {213.0, 16509839}, {214.0, 16509843}, {215.0, 16509845}, {216.0, 16509847}, {217.0, 16510361}, {218.0, 16510875}, {219.0, 16510879}, {220.0, 16510881}, {221.0, 16510883}, {222.0, 16511399}, {223.0, 16511911}, {224.0, 16511915}, {225.0, 16511917}, {226.0, 16511919}, {227.0, 16511923}, {228.0, 16512437}, {229.0, 16512951}, {230.0, 16512955}, {231.0, 16512957}, {232.0, 16512959}, {233.0, 16512961}, {234.0, 16512963}, {235.0, 16512967}, {236.0, 16513481}, {237.0, 16513995}, {238.0, 16513999}, {239.0, 16514001}, {240.0, 16514003}, {241.0, 16514005}, {242.0, 16514007}, {243.0, 16514011}, {244.0, 16514013}, {245.0, 16514015}, {246.0, 16514019}, {247.0, 16514021}, {248.0, 16514023}, {249.0, 16514027}, {250.0, 16514029}, {251.0, 16514031}, {252.0, 16514035}, {253.0, 16514037}, {254.0, 16514039}, {255.0, 16514043}] ("Z Scale.Marker Values[]")] -> w127
              tunnel: w124 -> [w130 w132 w134 w136 w138 w140 w142 w144 w146 w148 w150 w153]
              tunnel: [w130 w132 w134 w136 w138 w140 w142 w144 w146 w148 w150 w153] -> w128
              frame 0, Default {
                # "Fire"
              }
              frame 1 {
                # "Grayscale"
              }
              frame 2 {
                # "Red"
              }
              frame 3 {
                # "Green"
              }
              frame 4 {
                # "Blue"
              }
              frame 5 {
                # "Cyan"
              }
              frame 6 {
                # "Magenta"
              }
              frame 7 {
                # "Yellow"
              }
              frame 8 {
                # "Red-White"
              }
              frame 9 {
                # "Green-White"
              }
              frame 10 {
                # "Blue-White"
              }
              frame 11 {
              }
            }
            n83 = property class="IntGraph (strict)"(reference=w123, "ZScale.MarkerVals[]"=w127, "ZScale.High Color"=u32 255, "ZScale.Maximum"=w128) -> ()  [unwired: 1 in, 2 out]
          }
          frame 6 {
            w163 = u16 1 items=["Get Image", "Load and Read File"] ("Action")
            # "Shift Control Click - Open Image"
            n84 = call "OpenDBL.vi"("Action"=w163) -> ("Image"=w162:sgl[], "Dimensions (Z, Y, X, t)"=w161:i32[])  [unwired: 12 in, 1 out]
            n85 = Index Array(array=w161, index #1=1 ("index"), index #2=2 ("index")) -> (element #1=w158:i32, element #2=w156:i32)
            n86 = Reverse 1D Array(array=w162) -> (reversed array=w155:sgl[])
            n87 = Reshape Array(w155, w158, w156) -> (w157:sgl[][])
            n88 = Transpose 2D Array(2D array=w157) -> (transposed array=w154:sgl[][])
            n89 = property class="IntGraph (strict)"(reference=w164, "Value"=w154) -> ()  [unwired: 1 in, 2 out]
          }
          frame 4 {
            # "Control Click - Open for feature fitting"
            n90 = property class="IntGraph (strict)"(reference=w175) -> ("Value"=w169:sgl[][])  [unwired: 1 in, 2 out]
            n91 = local read "Image Acquisition Parameters"() -> (w168:T5)
            n92 = vi-ref "QuickProfile_V3.vi"() -> (w174:refnum<vi>)
            n93 = property class="VI Interface Type 5"(reference=w174) -> ("Path"=w171:path)  [unwired: 1 in, 2 out]
            n94 = Unbundle By Name(w168) -> ("Pixel Size (nm)"=w167:dbl[])
            n95 = Index Array(array=w167, index=0) -> (element=w165:dbl)
            n96 = Open VI Reference(type specifier VI Refnum (for type only)=w174, vi path=w171, options=128) -> (vi reference=w173:refnum<vi>)  [unwired: 3 in, 1 out]
            n97 = call-by-ref "Start Asynchronous Call"(reference=w173, "Image IN"=w169, "Pixel Size (nm)"=w165) -> (reference out=w170:refnum<vi>)  [unwired: 15 in, 1 out]
            n98 = Close Reference(reference=w170) -> ()  [unwired: 1 in, 1 out]
          }
          frame 10, Default {
            # "No match case"
          }
        }
      }
      event "Channel 1", "Channel 2", "Channel 3", "Channel 4", "Channel 5", "Channel 6": Mouse Up {
        n99 = event-data() -> ("CtlRef"=w178:refnum<vi>)  [unwired: 1 in]
        n100 = property class="IntGraph (strict)"(reference=w178) -> (reference out=w179:refnum<vi>, "ActPaletteTool"=w182:i32)  [unwired: 1 in, 1 out]
        n101 = Not Equal?(x=w182, y=0) -> (x != y?=w180:bool)
        n102 = case shown="True" w180 {
          tunnel: w179 -> [_ w186]
          tunnel: w176 -> [_ w183]
          frame False {
          }
          frame True {
            n103 = property class="IntGraph (strict)"(reference=w186) -> ("XScale.Range"=w185:T12, "YScale.Range"=w184:T12)  [unwired: 1 in, 2 out]
            n104 = for {
              tunnel: w185 -> [w188]
              tunnel: w184 -> [w189]
              tunnel: w183 -> [w187] mode=indexing
              n105 = property class="IntGraph (strict)"(reference=w187, "XScale.Range"=w188, "YScale.Range"=w189) -> ()  [unwired: 1 in, 2 out]
            }
          }
        }
      }
      event Timeout {
        n106 = event-data() -> ()  [unwired: 1 in, 3 out]
        n107 = Obtain Notifier(name (unnamed)="Running", notification data type=TRUE) -> (notifier out=w195:refnum<notifier>)  [unwired: 2 in, 2 out]
        n108 = Get Notifier Status(notifier=w195) -> (current notification=w193:bool)  [unwired: 1 in, 4 out]
        n109 = local read "Capture"() -> (w192:bool)
        n110 = And(x=w193, y=w192) -> (x .and. y?=w190:bool)
        n111 = case shown="False" w190 {
          tunnel: w191 -> [_ w199]
          frame False {
          }
          frame True {
            n112 = local write "Capture"(FALSE ("Capture")) -> ()
            n113 = Enqueue Element(queue=w199, element="Stop Acquisition" ("f")) -> ()  [unwired: 2 in, 3 out]
          }
        }
      }
      event Value Change {
        w218 = FALSE ("element")
        n114 = event-data() -> ()  [unwired: 1 in, 6 out]
        n115 = Unbundle By Name("Laser Controls") -> ("STED"=w224:bool, "640 nm"=w221:bool, "590 nm"=w222:bool, "485 nm"=w223:bool, "590 Power (V)"=w215:dbl, "STED Power (V)"=w214:dbl, "Manual Control"=w202:bool)
        n116 = local read "Live"() -> (w203:bool)
        n117 = Build Array(w224, w221, w222, w223, w218, w218, w218, w218) -> (w220:bool[])
        n118 = Or(x=w203, y=w202) -> (x .or. y?=w201:bool)
        n119 = Boolean Array To Number(Boolean array=w220) -> (number=w219:u32)
        n120 = case shown="True" w201 {
          tunnel: "Laser Controls" -> [_ w230]
          frame False {
          }
          frame True {
            n121 = call "FPGA-7842R-Control V1.vi"("Action"=FPGA-7842R-Reference."Laser Control", "Laser Controls"=w230, "Initialize"=TRUE) -> ()  [unwired: 12 in, 1 out]
          }
        }
        n122 = In Range and Coerce(upper limit=3.0, x=w215, lower limit=0.0) -> (coerced(x)=w209:dbl)  [unwired: 1 out]
        n123 = In Range and Coerce(upper limit=5.0, x=w214, lower limit=0.0) -> (coerced(x)=w208:dbl)  [unwired: 1 out]
        n124 = To Unsigned Byte Integer(number=w219) -> (unsigned 8bit integer=w217:u8)
        n125 = call "U8_To_U32.vi"("U8 IN"=w217) -> ("U32 OUT"=w216:u32)  [unwired: 13 in, 1 out]
        n126 = call "Volts to I16.vi"("Voltage (V)"=w209) -> ("I16"=w207:i16)  [unwired: 13 in, 1 out]
        n127 = call "Volts to I16.vi"("Voltage (V)"=w208) -> ("I16"=w206:i16)  [unwired: 13 in, 1 out]
        n128 = call "Scan Parameters Action Engine.vi"("Action"=enum16{"Read", "Write"}."Read") -> ("Scan Parameters OUT"=w227:T6)  [unwired: 14 in]
        n129 = Bundle By Name(cluster=w227, "Laser_States _U32"=w216, "590_Voltage_I16"=w207, "775_AOM_Volt_I16"=w206) -> (w225:T6)
        n130 = call "Scan Parameters Action Engine.vi"("Action"=enum16{"Read", "Write"}."Write", "Scan Parameters IN"=w225) -> ()  [unwired: 13 in, 1 out]
      }
      event "Dual Screens": Value Change {
        n131 = event-data() -> ("NewVal"=w234:bool)  [unwired: 1 in, 5 out]
        n132 = property class="App"() -> ("Disp.AllMonitors"=w235:T13)  [unwired: 2 in, 2 out]
        n133 = control-ref of="This VI"() -> (w233:refnum<vi>)
        n134 = case shown="False" w234 {
          tunnel: w235 -> [w238 w251]
          tunnel: T9 {"Left"=0, "Top"=0, "Right"=0, "Bottom"=0} ("FP Window Bounds 2") -> [w237 w250]
          tunnel: w233 -> [_ w249]
          frame False {
            w241 = i16 0
            n135 = Index Array(array=w238, index=0) -> (element=w245:T14)
            n136 = Unbundle By Name(w245) -> ("Bounds.Right"=w246:i16, "Bounds.Bottom"=w243:i16, "Bounds.Top"=w242:i16)
            n137 = Subtract(x=w243, y=w242) -> (x-y=w240:i16)
            n138 = Bundle By Name(cluster=w237, "Left"=w241, "Top"=w241, "Right"=w246, "Bottom"=w240) -> (w239:T9)
            n139 = property class="VI"("Front Panel.WinBounds"=w239) -> (reference out=w248:refnum<vi>)  [unwired: 2 in, 1 out]
            n140 = property class="VI"(reference=w248, "FP.State"=T10."Maximized" ("Front Panel Window:State")) -> ()  [unwired: 1 in, 2 out]
          }
          frame True {
            w260 = i16 0
            n141 = Index Array(array=w251, index #1=1 ("index"), index #2=0 ("index")) -> (element #1=w254:T14, element #2=w255:T14)
            n142 = Unbundle By Name(w254) -> ("Bounds.Right"=w256:i16)
            n143 = Unbundle By Name(w255) -> ("Bounds.Left"=w257:i16, "Bounds.Bottom"=w258:i16, "Bounds.Top"=w259:i16)
            n144 = Subtract(x=w256, y=w257) -> (x-y=w261:i16)
            n145 = Subtract(x=w258, y=w259) -> (x-y=w262:i16)
            n146 = Bundle By Name(cluster=w250, "Left"=w260, "Top"=w260, "Right"=w261, "Bottom"=w262) -> (w263:T9)
            n147 = property class="VI"(reference=w249, "Front Panel.WinBounds"=w263) -> ()  [unwired: 1 in, 2 out]
          }
        }
      }
      event Value Change {
        n148 = event-data() -> ("OldVal"=w283:T5, "NewVal"=w269:T5)  [unwired: 1 in]
        n149 = Equal?(x=w283, y=w269) -> (x = y?=w284:bool)
        n150 = case shown="False" w284 {
          tunnel: w269 -> [w286 _]
          tunnel: w283 -> [w296 _]
          frame False {
            n151 = Unbundle By Name(w286) -> ("Image Format"=w297:u16, "Scan Mode"=w289:enum16{"XY", "XZ", "YZ", "XYZ"})
            n152 = Unbundle By Name(w296) -> ("Scan Mode"=w290:enum16{"XY", "XZ", "YZ", "XYZ"})
            n153 = call "Scan Parameters Action Engine.vi"("Action"=enum16{"Read", "Write"}."Read") -> ("Scan Parameters OUT"=w292:T6)  [unwired: 14 in]
            n154 = Bundle By Name(cluster=w292, "Last_Scan_Mode"=w290, "Current_Scan_Mode"=w289) -> (w287:T6)
            n155 = case shown="\"XY\", Default" w290 {
              tunnel: w297 -> [w302 w330 w358 w386]
              tunnel: w297 -> [w301 w329 w357 w385]
              tunnel: w289 -> [w303 w331 w359 w387]
              tunnel: [w300 w328 w356 w384] -> w295
              tunnel: [w299 w327 w355 w383] -> w294
              tunnel: [w298 w326 w354 w382] -> w293
              frame "XY", Default {
                n156 = case shown="\"XZ\"" w303 {
                  tunnel: w302 -> [w305 w312 w317 w319]
                  tunnel: w301 -> [w306 w309 w316 w323]
                  tunnel: [w305 w308 w314 w320] -> w300
                  tunnel: [w306 w307 w313 w324] -> w299
                  tunnel: [FALSE ("Cursor.Visible") TRUE ("Cursor.Visible") TRUE ("Cursor.Visible") FALSE ("Cursor.Visible")] -> w298
                  frame "XY", Default {
                  }
                  frame "XZ" {
                    n157 = Increment(x=w309) -> (x+1=w308:u16)
                    n158 = Divide(x=w312, y=2) -> (x/y=w307:dbl)
                  }
                  frame "YZ" {
                    n159 = Increment(x=w317) -> (x+1=w313:u16)
                    n160 = Divide(x=w316, y=2) -> (x/y=w314:dbl)
                  }
                  frame "XYZ" {
                    n161 = Divide(x=w323, y=2) -> (x/y=w324:dbl)
                    n162 = Divide(x=w319, y=2) -> (x/y=w320:dbl)
                  }
                }
              }
              frame "XZ" {
                n163 = case shown="\"XYZ\"" w331 {
                  tunnel: w330 -> [w333 w340 w344 w347]
                  tunnel: w329 -> [w335 w339 w342 w351]
                  tunnel: [w332 w340 w341 w348] -> w328
                  tunnel: [w334 w339 w343 w352] -> w327
                  tunnel: [TRUE ("Cursor.Visible") FALSE ("Cursor.Visible") TRUE ("Cursor.Visible") FALSE ("Cursor.Visible")] -> w326
                  frame "XY" {
                    n164 = Increment(x=w333) -> (x+1=w332:u16)
                    n165 = Divide(x=w335, y=2) -> (x/y=w334:dbl)
                  }
                  frame "XZ", Default {
                  }
                  frame "YZ" {
                    n166 = Increment(x=w342) -> (x+1=w343:u16)
                    n167 = Divide(x=w344, y=2) -> (x/y=w341:dbl)
                  }
                  frame "XYZ" {
                    n168 = Divide(x=w351, y=2) -> (x/y=w352:dbl)
                    n169 = Divide(x=w347, y=2) -> (x/y=w348:dbl)
                  }
                }
              }
              frame "YZ" {
                n170 = case shown="\"YZ\", Default" w359 {
                  tunnel: w358 -> [w361 w369 w372 w380]
                  tunnel: w357 -> [w363 w367 w376 w381]
                  tunnel: [w360 w366 w373 w380] -> w356
                  tunnel: [w362 w368 w377 w381] -> w355
                  tunnel: [TRUE ("Cursor.Visible") TRUE ("Cursor.Visible") FALSE ("Cursor.Visible") FALSE ("Cursor.Visible")] -> w354
                  frame "XY" {
                    n171 = Increment(x=w361) -> (x+1=w360:u16)
                    n172 = Divide(x=w363, y=2) -> (x/y=w362:dbl)
                  }
                  frame "XZ" {
                    n173 = Increment(x=w367) -> (x+1=w368:u16)
                    n174 = Divide(x=w369, y=2) -> (x/y=w366:dbl)
                  }
                  frame "XYZ" {
                    n175 = Divide(x=w376, y=2) -> (x/y=w377:dbl)
                    n176 = Divide(x=w372, y=2) -> (x/y=w373:dbl)
                  }
                  frame "YZ", Default {
                  }
                }
              }
              frame "XYZ" {
                n177 = case shown="\"XYZ\", Default" w387 {
                  tunnel: w386 -> [w388 w400 w405 w408]
                  tunnel: w385 -> [w392 w395 w402 w409]
                  tunnel: [w389 w399 w404 w408] -> w384
                  tunnel: [w393 w396 w403 w409] -> w383
                  tunnel: [FALSE ("Cursor.Visible") TRUE ("Cursor.Visible") TRUE ("Cursor.Visible") FALSE ("Cursor.Visible")] -> w382
                  frame "XY" {
                    n178 = Divide(x=w392, y=2) -> (x/y=w393:dbl)
                    n179 = Divide(x=w388, y=2) -> (x/y=w389:dbl)
                  }
                  frame "XZ" {
                    n180 = Increment(x=w395) -> (x+1=w396:u16)
                    n181 = Divide(x=w400, y=2) -> (x/y=w399:dbl)
                  }
                  frame "YZ" {
                    n182 = Increment(x=w405) -> (x+1=w404:u16)
                    n183 = Divide(x=w402, y=2) -> (x/y=w403:dbl)
                  }
                  frame "XYZ", Default {
                  }
                }
              }
            }
            n184 = property on="Channel 1" class="IntGraph (strict)"("Cursor.Cursor X"=w295, "Cursor.Cursor Y"=w294, "Cursor.Visible"=w293) -> ()  [unwired: 2 in, 2 out]
            n185 = call "Scan Parameters Action Engine.vi"("Action"=enum16{"Read", "Write"}."Write", "Scan Parameters IN"=w287) -> ()  [unwired: 13 in, 1 out]
          }
          frame True {
            n186 = property on="Channel 1" class="IntGraph (strict)"("Cursor.Visible"=FALSE) -> ()  [unwired: 2 in, 2 out]
          }
        }
        n187 = Unbundle By Name(w269) -> ("Image Dimension (um)"=w270:dbl[], "Scan Type"=w275:enum16{"Sample Scanning", "Beam Scanning"})
        n188 = Equal?(x=w275, y=enum16{"Sample Scanning", "Beam Scanning"}."Beam Scanning") -> (x = y?=w277:bool)
        n189 = Index Array(array=w270, index=0) -> (element=w278:dbl)
        n190 = call "Res Mirror um to Volts.vi"("Image Size (um)"=w278) -> ("Voltage (V)"=w279:dbl)
        n191 = In Range and Coerce(upper limit=4.8, x=w279, lower limit=0.0) -> (coerced(x)=w280:dbl)  [unwired: 1 out]
        n192 = call "Volts to I16.vi"("Voltage (V)"=w280) -> ("I16"=w274:i16)  [unwired: 13 in, 1 out]
        n193 = call "Manual Controls Action Engine.vi"("Action"=enum16{"Read", "Write"}."Read") -> ("Manual Controls Out"=w267:T1)  [unwired: 14 in]
        n194 = Bundle By Name(cluster=w267, "Res Mirror Amp (I16)"=w274, "Res Mirror Mute"=w277) -> (w265:T1)
        n195 = call "Manual Controls Action Engine.vi"("Action"=enum16{"Read", "Write"}."Write", "Manual Controls In"=w265) -> ("Manual Controls Out"=w264:T1)  [unwired: 13 in]
        n196 = call "FPGA-7842R-Control V1.vi"("Action"=FPGA-7842R-Reference."Set Res Mirror", "Manual Controls"=w264, "Initialize"=TRUE) -> ()  [unwired: 12 in, 1 out]
      }
      event "Unused Axis Voltage": Value Change {
        n197 = event-data() -> ()  [unwired: 1 in, 6 out]
        n198 = call "FPGA-7842R-Control V1.vi"("Action"=FPGA-7842R-Reference."Unused Axis I16", "Initialize"=TRUE, "Unused Axis Offset (I16)"="Unused Axis Voltage") -> ()  [unwired: 12 in, 1 out]
      }
      event Value Change {
        n199 = event-data() -> ("OldVal"=w428:T2, "NewVal"=w427:T2)  [unwired: 1 in, 4 out]
        n200 = property on="Stage Control" class="Clust"() -> ("Controls[]"=w429:refnum<vi>[])  [unwired: 2 in, 2 out]
        n201 = Not Equal?(x=w428, y=w427) -> (x != y?=w426:T15)
        n202 = Unbundle By Name(w427) -> ("Mode"=w421:enum32{"Joystick", "Coarse", "Fine"}, "Step Size (um)"=w420:T16, "Velocity"=w418:enum16{"Low", "Medium", "High"})
        n203 = Cluster To Array(cluster=w426) -> (array=w425:bool[])
        n204 = for {
          tunnel: w429 -> [w437] mode=indexing
          tunnel: w425 -> [w438] mode=indexing
          tunnel: [w437] -> w430
          stop <- w438 stop-if-true
        }
        n205 = Format Into String(w418) -> (resulting string=w417:string)  [unwired: 3 in, 1 out]
        n206 = Format Into String(w420) -> (resulting string=w422:string)  [unwired: 3 in, 1 out]
        n207 = case shown="\"High\"" w417 {
          tunnel: [0.5 1.0 0.0] -> w416
          frame "Medium", Default {
          }
          frame "High" {
          }
          frame "Low" {
          }
        }
        n208 = property class="Ctl"(reference=w430) -> ("ClassName"=w431:string, "Label.Text"=w432:string)  [unwired: 1 in, 2 out]
        n209 = control-ref of="Halt"() -> (w423:refnum<vi>)
        n210 = Fract/Exp String To Number(string=w422) -> (number=w419:dbl)  [unwired: 3 in, 1 out]
        n211 = case shown="\"Fine\"" w421 {
          tunnel: w424 -> [w446 w457 w530 w539]
          tunnel: w431 -> [_ w456 _ w538]
          tunnel: w432 -> [_ w455 _ w537]
          tunnel: [w441 w451 w529 w534] -> w433
          tunnel: w423 -> [w440 w450 w528 w533]
          tunnel: w419 -> [_ w449 _ w532]
          tunnel: w416 -> [w439 w448 _ _]
          frame "Joystick" {
            w445 = TRUE
            n212 = Build Array(w445, w445) -> (w444:bool[])
            n213 = call "M686.vi"("Velocity"=w439, "Abort"=w440, "Axis"=w444, "Action"=StageStates."JOYSTICK", "VISA In"=w446) -> ("VISA Out"=w443:refnum<visa-resource-name>)  [unwired: 3 in, 3 out]
            n214 = call "M686.vi"("Abort"=w440, "Action"=StageStates."POSITION", "VISA In"=w443) -> ("Position Out"=w441:dbl[])  [unwired: 5 in, 3 out]
          }
          frame "Coarse" {
            w459 = FALSE
            n215 = Build Array(w459, w459) -> (w458:bool[])
            n216 = call "M686.vi"("Abort"=w450, "Axis"=w458, "Action"=StageStates."JOYSTICK", "VISA In"=w457) -> ("VISA Out"=w454:refnum<visa-resource-name>)  [unwired: 4 in, 3 out]
            n217 = Divide(x=w449, y=1000.0) -> (x/y=w453:dbl)
            n218 = case shown="\"Boolean\"" w456 {
              tunnel: w455 -> [_ w470]
              tunnel: w454 -> [w464 w469]
              tunnel: w453 -> [_ w468]
              tunnel: w450 -> [w461 w467]
              tunnel: [w463 w466] -> w451
              tunnel: w448 -> [_ w465]
              frame Default {
                n219 = call "M686.vi"("Abort"=w461, "Action"=StageStates."POSITION", "VISA In"=w464) -> ("Position Out"=w463:dbl[])  [unwired: 5 in, 3 out]
              }
              frame "Boolean" {
                n220 = case shown="\"Right\"" w470 {
                  tunnel: w469 -> [_ w475 w482 w495 w506 w517 w527]
                  tunnel: w468 -> [_ _ _ w493 w504 w515 w521]
                  tunnel: w467 -> [_ w473 w480 w488 w498 w509 w520]
                  tunnel: [dbl[] [] ("Position Out") w472 w479 w487 w497 w508 w519] -> w466
                  tunnel: w465 -> [_ _ _ w486 w496 w507 w518]
                  frame Default {
                  }
                  frame "Home" {
                    w477 = TRUE
                    n221 = Build Array(w477, w477) -> (w478:bool[])
                    n222 = call "M686.vi"("Velocity"=1.0, "Abort"=w473, "Axis"=w478, "Action"=StageStates."HOME", "VISA In"=w475) -> ("Position Out"=w472:dbl[])  [unwired: 3 in, 3 out]
                  }
                  frame "Halt" {
                    w484 = TRUE
                    n223 = Build Array(w484, w484) -> (w485:bool[])
                    n224 = call "M686.vi"("Velocity"=1.0, "Abort"=w480, "Axis"=w485, "Action"=StageStates."HALT", "VISA In"=w482) -> ("Position Out"=w479:dbl[])  [unwired: 3 in, 3 out]
                  }
                  frame "Up" {
                    n225 = Build Array(w493, w493) -> (w492:dbl[])
                    n226 = Build Array(FALSE, TRUE) -> (w489:bool[])
                    n227 = call "M686.vi"("Velocity"=w486, "Abort"=w488, "Axis"=w489, "Positions"=w492, "Action"=StageStates."MVR", "VISA In"=w495) -> ("Position Out"=w487:dbl[])  [unwired: 2 in, 3 out]
                  }
                  frame "Down" {
                    n228 = Negate(x=w504) -> (-x=w499:dbl)
                    n229 = Build Array(w499, w499) -> (w503:dbl[])
                    n230 = Build Array(FALSE, TRUE) -> (w500:bool[])
                    n231 = call "M686.vi"("Velocity"=w496, "Abort"=w498, "Axis"=w500, "Positions"=w503, "Action"=StageStates."MVR", "VISA In"=w506) -> ("Position Out"=w497:dbl[])  [unwired: 2 in, 3 out]
                  }
                  frame "Left" {
                    n232 = Negate(x=w515) -> (-x=w510:dbl)
                    n233 = Build Array(w510, w510) -> (w514:dbl[])
                    n234 = Build Array(TRUE, FALSE) -> (w511:bool[])
                    n235 = call "M686.vi"("Velocity"=w507, "Abort"=w509, "Axis"=w511, "Positions"=w514, "Action"=StageStates."MVR", "VISA In"=w517) -> ("Position Out"=w508:dbl[])  [unwired: 2 in, 3 out]
                  }
                  frame "Right" {
                    n236 = Build Array(w521, w521) -> (w525:dbl[])
                    n237 = Build Array(TRUE, FALSE) -> (w522:bool[])
                    n238 = call "M686.vi"("Velocity"=w518, "Abort"=w520, "Axis"=w522, "Positions"=w525, "Action"=StageStates."MVR", "VISA In"=w527) -> ("Position Out"=w519:dbl[])  [unwired: 2 in, 3 out]
                  }
                }
              }
            }
          }
          frame Default {
            n239 = call "M686.vi"("Abort"=w528, "Action"=StageStates."POSITION", "VISA In"=w530) -> ("Position Out"=w529:dbl[])  [unwired: 5 in, 3 out]
          }
          frame "Fine" {
            w541 = FALSE
            n240 = case shown="\"Boolean\"" w538 {
              tunnel: w537 -> [_ w552]
              tunnel: w532 -> [_ w551]
              frame "False", Default {
              }
              frame "Boolean" {
                n241 = call "Manual Controls Action Engine.vi"("Action"=enum16{"Read", "Write"}."Read") -> ("Manual Controls Out"=w544:T1)  [unwired: 14 in]
                n242 = call "Scanning Volts to Microns.vi"() -> ("Scanning Conversions OUT"=w550:T17)
                n243 = case shown="\"Down\"" w552 {
                  tunnel: w551 -> [_ w560 _ w573 w582 w591]
                  tunnel: w550 -> [_ w562 _ w575 w584 w593]
                  tunnel: w544 -> [w553 w558 w566 w571 w580 w589]
                  tunnel: [w553 w557 w565 w570 w579 w588] -> w543
                  frame Default {
                  }
                  frame "Up" {
                    n244 = Unbundle By Name(w562) -> ("Stage Y Axis (Volts/um)"=w561:dbl)
                    n245 = Unbundle By Name(w558) -> ("Y Axis Voltage (I16)"=w559:i16)
                    n246 = Multiply(x=w560, y=w561) -> (x*y=w555:dbl)
                    n247 = call "Volts to I16.vi"("Voltage (V)"=w555) -> ("I16"=w554:i16)  [unwired: 13 in, 1 out]
                    n248 = Add(x=w559, y=w554) -> (x+y=w556:i16)
                    n249 = Bundle By Name(cluster=w558, "Y Axis Voltage (I16)"=w556) -> (w557:T1)
                  }
                  frame "Home" {
                    n250 = call "Volts to I16.vi"("Voltage (V)"=5.0 ("Stage Y Axis Offset (V)")) -> ("I16"=w563:i16)  [unwired: 13 in, 1 out]
                    n251 = Bundle By Name(cluster=w566, "X Axis Voltage (I16)"=w563, "Y Axis Voltage (I16)"=w563, "Z Axis Voltage (I16)"=w563) -> (w565:T1)
                  }
                  frame "Down" {
                    n252 = Unbundle By Name(w571) -> ("Y Axis Voltage (I16)"=w572:i16)
                    n253 = Unbundle By Name(w575) -> ("Stage Y Axis (Volts/um)"=w574:dbl)
                    n254 = Multiply(x=w573, y=w574) -> (x*y=w568:dbl)
                    n255 = call "Volts to I16.vi"("Voltage (V)"=w568) -> ("I16"=w567:i16)  [unwired: 13 in, 1 out]
                    n256 = Subtract(x=w572, y=w567) -> (x-y=w569:i16)
                    n257 = Bundle By Name(cluster=w571, "Y Axis Voltage (I16)"=w569) -> (w570:T1)
                  }
                  frame "Left" {
                    n258 = Unbundle By Name(w584) -> ("Stage X Axis (Volts/um)"=w583:dbl)
                    n259 = Unbundle By Name(w580) -> ("X Axis Voltage (I16)"=w581:i16)
                    n260 = Multiply(x=w582, y=w583) -> (x*y=w577:dbl)
                    n261 = call "Volts to I16.vi"("Voltage (V)"=w577) -> ("I16"=w576:i16)  [unwired: 13 in, 1 out]
                    n262 = Subtract(x=w581, y=w576) -> (x-y=w578:i16)
                    n263 = Bundle By Name(cluster=w580, "X Axis Voltage (I16)"=w578) -> (w579:T1)
                  }
                  frame "Right" {
                    n264 = Unbundle By Name(w593) -> ("Stage X Axis (Volts/um)"=w592:dbl)
                    n265 = Unbundle By Name(w589) -> ("X Axis Voltage (I16)"=w590:i16)
                    n266 = Multiply(x=w591, y=w592) -> (x*y=w586:dbl)
                    n267 = call "Volts to I16.vi"("Voltage (V)"=w586) -> ("I16"=w585:i16)  [unwired: 13 in, 1 out]
                    n268 = Add(x=w590, y=w585) -> (x+y=w587:i16)
                    n269 = Bundle By Name(cluster=w589, "X Axis Voltage (I16)"=w587) -> (w588:T1)
                  }
                }
                n270 = call "Manual Controls Action Engine.vi"("Action"=enum16{"Read", "Write"}."Write", "Manual Controls In"=w543) -> ("Manual Controls Out"=w547:T1)  [unwired: 13 in]
                n271 = call "FPGA-7842R-Control V1.vi"("Action"=FPGA-7842R-Reference."Stage Control", "Manual Controls"=w547, "Initialize"=TRUE) -> ()  [unwired: 12 in, 1 out]
              }
            }
            n272 = Build Array(w541, w541) -> (w540:bool[])
            n273 = call "M686.vi"("Abort"=w533, "Axis"=w540, "Action"=StageStates."JOYSTICK", "VISA In"=w539) -> ("VISA Out"=w536:refnum<visa-resource-name>)  [unwired: 4 in, 3 out]
            n274 = call "M686.vi"("Abort"=w533, "Action"=StageStates."POSITION", "VISA In"=w536) -> ("Position Out"=w534:dbl[])  [unwired: 5 in, 3 out]
          }
        }
        n275 = Index Array(array=w433) -> ()  [unwired: 2 in, 2 out]
      }
      event "Set Mode Offset": Value Change {
        n276 = event-data() -> ("NewVal"=w594:bool)  [unwired: 1 in]
        n277 = case shown="True" w594 {
          frame False {
          }
          frame True {
            # "Vert Pixels"
            # "Horz Pixels"
            # "Z Pixel Size"
            # "XY Pixel Size"
            # "Z volts per um"
            # "XY volts per um"
            n278 = local read "Image Acquisition Parameters"() -> (w609:T5)
            n279 = Unbundle By Name(w609) -> ("Image Format"=w610:u16, "Image Dimension (um)"=w613:dbl[])
            n280 = call "Scanning Volts to Microns.vi"() -> ("Scanning Conversions OUT"=w598:T17)
            n281 = Unbundle By Name(w598) -> ("Stage X Axis (Volts/um)"=w597:dbl, "Stage Z Axis (Volts/um)"=w596:dbl)
            n282 = property on="Channel 1" class="IntGraph (strict)"() -> ("Cursor.Cursor X"=w604:dbl, "Cursor.Cursor Y"=w605:dbl)  [unwired: 2 in, 2 out]
            n283 = To Double Precision Float(number=w610) -> (double precision float=w601:dbl)
            n284 = call "Scan Parameters Action Engine.vi"("Action"=enum16{"Read", "Write"}."Read") -> ("Scan Parameters OUT"=w618:T6)  [unwired: 14 in]
            n285 = Divide(x=w613, y=w601) -> (x/y=w614:dbl[])
            n286 = Unbundle By Name(w618) -> ("Last_Scan_Mode"=w607:enum16{"XY", "XZ", "YZ", "XYZ"}, "Current_Scan_Mode"=w608:enum16{"XY", "XZ", "YZ", "XYZ"})
            n287 = Index Array(array=w614, index #1=0 ("index"), index #2=1 ("index")) -> (element #1=w615:dbl, element #2=w616:dbl)
            n288 = Divide(x=w601, y=2.0) -> (x/y=w600:dbl)
            n289 = case shown="\"XY\", Default" w607 {
              tunnel: w608 -> [w623 w686 w733 w780]
              tunnel: w604 -> [w624 w678 w725 w772]
              tunnel: w605 -> [w625 w679 w726 w773]
              tunnel: w600 -> [w631 w685 w732 w779]
              tunnel: w615 -> [w630 w684 w731 w778]
              tunnel: w596 -> [w628 w682 w729 w776]
              tunnel: w597 -> [w629 w683 w730 w777]
              tunnel: w616 -> [w627 w681 w728 w775]
              tunnel: w600 -> [w626 w680 w727 w774]
              tunnel: w618 -> [w622 w677 w724 w771]
              tunnel: [w621 w676 w723 w770] -> w619
              tunnel: [w620 w675 w722 w769] -> w603
              frame "XY", Default {
                # "XY Scan Mode"
                n290 = case shown="\"YZ\"" w623 {
                  tunnel: w631 -> [w640 _ w666 _]
                  tunnel: w630 -> [w642 w660 w671 _]
                  tunnel: w629 -> [w641 w658 w669 _]
                  tunnel: w628 -> [_ _ _ _]
                  tunnel: w627 -> [_ _ _ _]
                  tunnel: w626 -> [w638 w656 _ _]
                  tunnel: w625 -> [w639 w655 _ _]
                  tunnel: w624 -> [w647 _ w665 _]
                  tunnel: w622 -> [w646 w652 w664 w674]
                  tunnel: [w645 w653 w663 w674] -> w621
                  tunnel: [w650 w651 w662 w673] -> w620
                  frame "XY", Default {
                    # "XY - No change"
                    n291 = Unbundle By Name(w646) -> ("Stage_X_Off_V"=w636:dbl, "Stage_Y_Off_V"=w634:dbl, "Stage_Z_Off_V"=w650:dbl)
                    n292 = Subtract(x=w647, y=w640) -> (x-y=w649:dbl)
                    n293 = Multiply(x=w649, y=w642) -> (x*y=w648:dbl)
                    n294 = Multiply(x=w648, y=w641) -> (x*y=w637:dbl)
                    n295 = Subtract(x=w639, y=w638) -> (x-y=w643:dbl)
                    n296 = Multiply(x=w643, y=w642) -> (x*y=w644:dbl)
                    n297 = Add(x=w636, y=w637) -> (x+y=w635:dbl)
                    n298 = Multiply(x=w644, y=w641) -> (x*y=w633:dbl)
                    n299 = Add(x=w634, y=w633) -> (x+y=w632:dbl)
                    n300 = Bundle By Name(cluster=w646, "Stage_X_Off_V"=w635, "Stage_Y_Off_V"=w632) -> (w645:T6)
                  }
                  frame "XZ" {
                    # "XZ - Grab Y cusor position - Set Y offset"
                    n301 = Subtract(x=w655, y=w656) -> (x-y=w661:dbl)
                    n302 = Unbundle By Name(w652) -> ("Stage_Y_Off_V"=w654:dbl)
                    n303 = Multiply(x=w661, y=w660) -> (x*y=w659:dbl)
                    n304 = Multiply(x=w659, y=w658) -> (x*y=w657:dbl)
                    n305 = Add(x=w654, y=w657) -> (x+y=w651:dbl)
                    n306 = Bundle By Name(cluster=w652, "Stage_Y_Off_V"=w651) -> (w653:T6)
                  }
                  frame "YZ" {
                    # "YZ - Grab X cursor position - Set X offset"
                    n307 = Subtract(x=w665, y=w666) -> (x-y=w672:dbl)
                    n308 = Unbundle By Name(w664) -> ("Stage_X_Off_V"=w668:dbl)
                    n309 = Multiply(x=w672, y=w671) -> (x*y=w670:dbl)
                    n310 = Multiply(x=w670, y=w669) -> (x*y=w667:dbl)
                    n311 = Add(x=w668, y=w667) -> (x+y=w662:dbl)
                    n312 = Bundle By Name(cluster=w664, "Stage_X_Off_V"=w662) -> (w663:T6)
                  }
                  frame "XYZ" {
                    # "XYZ - No change"
                    n313 = Unbundle By Name(w674) -> ("Stage_Z_Off_V"=w673:dbl)
                  }
                }
              }
              frame "XZ" {
                # "XZ Scan Mode"
                n314 = case shown="\"YZ\"" w686 {
                  tunnel: w685 -> [_ _ w702 _]
                  tunnel: w684 -> [_ _ w709 _]
                  tunnel: w683 -> [_ _ w706 _]
                  tunnel: w682 -> [w689 _ _ w713]
                  tunnel: w677 -> [w696 w699 w708 w720]
                  tunnel: w681 -> [w688 _ _ w712]
                  tunnel: [w693 w699 w703 w717] -> w676
                  tunnel: w680 -> [w692 _ _ w716]
                  tunnel: w679 -> [w691 _ _ w715]
                  tunnel: w678 -> [_ _ w701 _]
                  tunnel: [w687 w698 w700 w711] -> w675
                  frame "XY", Default {
                    # "XY - Grab Y cusor position - Set Z offset"
                    n315 = Subtract(x=w691, y=w692) -> (x-y=w697:dbl)
                    n316 = Unbundle By Name(w696) -> ("Stage_Z_Off_V"=w690:dbl)
                    n317 = Multiply(x=w697, y=w688) -> (x*y=w695:dbl)
                    n318 = Multiply(x=w695, y=w689) -> (x*y=w694:dbl)
                    n319 = Add(x=w690, y=w694) -> (x+y=w687:dbl)
                    n320 = Bundle By Name(cluster=w696, "Stage_Z_Off_V"=w687) -> (w693:T6)
                  }
                  frame "XZ" {
                    # "XZ - No change"
                    n321 = Unbundle By Name(w699) -> ("Stage_Z_Off_V"=w698:dbl)
                  }
                  frame "YZ" {
                    # "YZ - Grab X cursor position - Set X offset"
                    n322 = Subtract(x=w701, y=w702) -> (x-y=w710:dbl)
                    n323 = Unbundle By Name(w708) -> ("Stage_X_Off_V"=w705:dbl)
                    n324 = Multiply(x=w710, y=w709) -> (x*y=w707:dbl)
                    n325 = Multiply(x=w707, y=w706) -> (x*y=w704:dbl)
                    n326 = Add(x=w705, y=w704) -> (x+y=w700:dbl)
                    n327 = Bundle By Name(cluster=w708, "Stage_X_Off_V"=w700) -> (w703:T6)
                  }
                  frame "XYZ" {
                    # "XYZ - Grab Y cusor position - Set Z offset"
                    n328 = Subtract(x=w715, y=w716) -> (x-y=w721:dbl)
                    n329 = Unbundle By Name(w720) -> ("Stage_Z_Off_V"=w714:dbl)
                    n330 = Multiply(x=w721, y=w712) -> (x*y=w719:dbl)
                    n331 = Multiply(x=w719, y=w713) -> (x*y=w718:dbl)
                    n332 = Add(x=w714, y=w718) -> (x+y=w711:dbl)
                    n333 = Bundle By Name(cluster=w720, "Stage_Z_Off_V"=w711) -> (w717:T6)
                  }
                }
              }
              frame "YZ" {
                # "YZ Scan Mode"
                n334 = case shown="\"XZ\"" w733 {
                  tunnel: w732 -> [_ w747 _ _]
                  tunnel: w731 -> [_ w754 _ _]
                  tunnel: w730 -> [_ w751 _ _]
                  tunnel: w729 -> [w736 _ _ w760]
                  tunnel: w724 -> [w743 w753 w757 w767]
                  tunnel: w728 -> [w735 _ _ w759]
                  tunnel: [w740 w748 w757 w764] -> w723
                  tunnel: w727 -> [w739 _ _ w763]
                  tunnel: w726 -> [w738 _ _ w762]
                  tunnel: w725 -> [_ w746 _ _]
                  tunnel: [w734 w745 w756 w758] -> w722
                  frame "XY", Default {
                    # "XY - Grab Y cusor position - Set Z offset"
                    n335 = Subtract(x=w738, y=w739) -> (x-y=w744:dbl)
                    n336 = Unbundle By Name(w743) -> ("Stage_Z_Off_V"=w737:dbl)
                    n337 = Multiply(x=w744, y=w735) -> (x*y=w742:dbl)
                    n338 = Multiply(x=w742, y=w736) -> (x*y=w741:dbl)
                    n339 = Add(x=w737, y=w741) -> (x+y=w734:dbl)
                    n340 = Bundle By Name(cluster=w743, "Stage_Z_Off_V"=w734) -> (w740:T6)
                  }
                  frame "XZ" {
                    # "XZ - Grab X cursor position - Set Y offset"
                    n341 = Subtract(x=w746, y=w747) -> (x-y=w755:dbl)
                    n342 = Unbundle By Name(w753) -> ("Stage_Y_Off_V"=w750:dbl)
                    n343 = Multiply(x=w755, y=w754) -> (x*y=w752:dbl)
                    n344 = Multiply(x=w752, y=w751) -> (x*y=w749:dbl)
                    n345 = Add(x=w750, y=w749) -> (x+y=w745:dbl)
                    n346 = Bundle By Name(cluster=w753, "Stage_Y_Off_V"=w745) -> (w748:T6)
                  }
                  frame "YZ" {
                    # "YZ - No change"
                    n347 = Unbundle By Name(w757) -> ("Stage_Z_Off_V"=w756:dbl)
                  }
                  frame "XYZ" {
                    # "XYZ - Grab Y cusor position - Set Z offset"
                    n348 = Subtract(x=w762, y=w763) -> (x-y=w768:dbl)
                    n349 = Unbundle By Name(w767) -> ("Stage_Z_Off_V"=w761:dbl)
                    n350 = Multiply(x=w768, y=w759) -> (x*y=w766:dbl)
                    n351 = Multiply(x=w766, y=w760) -> (x*y=w765:dbl)
                    n352 = Add(x=w761, y=w765) -> (x+y=w758:dbl)
                    n353 = Bundle By Name(cluster=w767, "Stage_Z_Off_V"=w758) -> (w764:T6)
                  }
                }
              }
              frame "XYZ" {
                # "XYZ Scan Mode"
                n354 = case shown="\"XZ\"" w780 {
                  tunnel: w779 -> [_ _ w796 _]
                  tunnel: w778 -> [_ w792 w803 _]
                  tunnel: w777 -> [_ w789 w800 _]
                  tunnel: w776 -> [_ _ _ _]
                  tunnel: w771 -> [w782 w791 w802 w806]
                  tunnel: w775 -> [_ _ _ _]
                  tunnel: [w782 w787 w797 w806] -> w770
                  tunnel: w774 -> [_ w786 _ _]
                  tunnel: w773 -> [_ w785 _ _]
                  tunnel: w772 -> [_ _ w795 _]
                  tunnel: [w781 w783 w794 w805] -> w769
                  frame "XY", Default {
                    # "XY - No change"
                    n355 = Unbundle By Name(w782) -> ("Stage_Z_Off_V"=w781:dbl)
                  }
                  frame "XZ" {
                    # "XZ - Grab Y cusor position - Set Y offset"
                    n356 = Subtract(x=w785, y=w786) -> (x-y=w793:dbl)
                    n357 = Unbundle By Name(w791) -> ("Stage_Y_Off_V"=w784:dbl)
                    n358 = Multiply(x=w793, y=w792) -> (x*y=w790:dbl)
                    n359 = Multiply(x=w790, y=w789) -> (x*y=w788:dbl)
                    n360 = Add(x=w784, y=w788) -> (x+y=w783:dbl)
                    n361 = Bundle By Name(cluster=w791, "Stage_Y_Off_V"=w783) -> (w787:T6)
                  }
                  frame "YZ" {
                    # "YZ - Grab X cursor position - Set X offset"
                    n362 = Subtract(x=w795, y=w796) -> (x-y=w804:dbl)
                    n363 = Unbundle By Name(w802) -> ("Stage_X_Off_V"=w799:dbl)
                    n364 = Multiply(x=w804, y=w803) -> (x*y=w801:dbl)
                    n365 = Multiply(x=w801, y=w800) -> (x*y=w798:dbl)
                    n366 = Add(x=w799, y=w798) -> (x+y=w794:dbl)
                    n367 = Bundle By Name(cluster=w802, "Stage_X_Off_V"=w794) -> (w797:T6)
                  }
                  frame "XYZ" {
                    # "XYZ - No change"
                    n368 = Unbundle By Name(w806) -> ("Stage_Z_Off_V"=w805:dbl)
                  }
                }
              }
            }
            n369 = call "Volts to I16.vi"("Voltage (V)"=w603) -> ("I16"=w602:i16)  [unwired: 13 in, 1 out]
            n370 = local write "Unused Axis Voltage"(w602) -> ()
            n371 = call "Scan Parameters Action Engine.vi"("Action"=enum16{"Read", "Write"}."Write", "Scan Parameters IN"=w619) -> ()  [unwired: 13 in, 1 out]
          }
        }
      }
      event "show cursor": Value Change {
        w808 = 50.0 ("Cursor.Cursor Position:Cursor X")
        n372 = event-data() -> ("NewVal"=w809:bool)  [unwired: 1 in, 5 out]
        n373 = property on="Channel 1" class="IntGraph (strict)"("Cursor.Cursor X"=w808, "Cursor.Cursor Y"=w808, "Cursor.Visible"=w809) -> ()  [unwired: 2 in, 2 out]
      }
    }
  }
  n374 = while {
    shift-right: [w818] -> _
    shift-left: "Idle" -> [w819]
    tunnel: w16 -> [w815]
    shift-right: [w813] -> _
    shift-left: w13 -> [w814]
    tunnel: w4 -> [w810]
    stop <- w817 stop-if-true
    n375 = case shown="\"Start Waveforms\"" w819 {
      selector: w819 -> [_ _ _ w849 _ _ _ _ _ _]
      tunnel: ["Exit" w826 "Idle" ("name (unnamed)") "Arange Displays" ("name (unnamed)") "Start FPGA Acquisition" ("name (unnamed)") "Display" ("name (unnamed)") "Close Images" ("name (unnamed)") "Idle" "Stop Waveforms" ("name (unnamed)") "Start Waveforms" ("name (unnamed)")] -> w818
      tunnel: [TRUE w828 w835 w857 w871 w883 w919 w952 w957 w963] -> w817
      tunnel: FALSE -> [_ w828 w835 w857 w871 w883 w919 w952 w957 w963]
      tunnel: w815 -> [_ w827 _ _ _ _ _ _ _ _]
      tunnel: w814 -> [w822 w825 w836 w855 w868 w881 w917 w950 w958 w964]
      tunnel: [w821 w825 w836 w855 w868 w876 w917 w949 w958 w964] -> w813
      tunnel: "Image Acquisition Parameters" -> [_ _ _ w848 _ w873 _ _ _ w961]
      tunnel: "Detectors" -> [_ _ _ w847 _ _ _ _ _ w959]
      tunnel: w810 -> [_ _ _ _ w864 _ _ _ _ _]
      frame "Exit" {
        n376 = call "FPGA-7842R-Control V1.vi"("Action"=FPGA-7842R-Reference."Close FPGA", "Initialize"=w822) -> ("Initalized"=w821:bool)  [unwired: 13 in]
      }
      frame "Idle", Default {
        n377 = Dequeue Element(queue=w827, timeout in ms (-1)=-1) -> (element=w826:string)  [unwired: 1 in, 3 out]
      }
      frame "Close Images" {
        w831 = u16 0 items=["Read", "Write"] ("Mode")
        w832 = u16 0 items=["Write", "Read"] ("Mode")
        n378 = call "File Action V1.vi"("Mode"=w831) -> ("Files Open"=w830:bool)  [unwired: 12 in, 2 out]
        n379 = call "Image_Actions_V1.vi"("Mode"=w832, "Action"="Trash Images") -> ()  [unwired: 12 in, 2 out]
        n380 = case shown="True" w830 {
          frame False {
          }
          frame True {
            w838 = u16 1 items=["Read", "Write"] ("Mode")
            n381 = call "File Action V1.vi"("Action"="Close Files", "Mode"=w838) -> ()  [unwired: 11 in, 3 out]
          }
        }
      }
      frame "Capture", "Live" {
        w853 = u16 0 items=["Write", "Read"] ("Mode")
        n382 = Cluster To Array(cluster=w847) -> (array=w845:bool[])
        n383 = Index Array(array=w845, index=4) -> (element=w842:bool)
        n384 = Boolean To (0,1)(Boolean=w845) -> (0, 1=w846:i16[])
        n385 = Add Array Elements(numeric array=w846) -> (sum=w843:i16)
        n386 = To Long Integer(number=w843) -> (32bit integer=w840:i32)
        n387 = Unbundle By Name(w848) -> ("Image Format"=w850:u16)
        n388 = Select(t=1, s=w842, f=w840) -> (s? t:f=w839:i32)
        n389 = case shown="Default" w849 {
          tunnel: w848 -> [_ w859]
          tunnel: w839 -> [_ w858]
          frame Default {
          }
          frame "Capture" {
            w862 = u16 1 items=["Read", "Write"] ("Mode")
            n390 = call "File Action V1.vi"("Action"="Open Files", "Mode"=w862, "Image Acquisition Parameters"=w859, "File Path IN"="Save File Path", "Number of Channels"=w858) -> ("File Path OUT"=w860:path)  [unwired: 8 in, 2 out]
            n391 = local write "Save File Path"(w860) -> ()
          }
        }
        n392 = To Long Integer(number=w850) -> (32bit integer=w852:i32)
        n393 = Bundle(w852, w852) -> (w851:cluster{i32, i32})  [unwired: 1 in]
        n394 = call "Image_Actions_V1.vi"("Image Size (Pixels)"=w851, "Mode"=w853, "Number of Channels"=w839, "Action"="Create Images") -> ()  [unwired: 10 in, 2 out]
      }
      frame "Arange Displays" {
        w866 = u16 1 items=["Write", "Read"] ("Mode")
        w870 = 1.0  # Aspect Ratio (h/w)
        w869 = u16 1 items=["Read", "Write"] ("Action")
        n395 = call "Image_Actions_V1.vi"("Mode"=w866) -> ("Image REFs OUT"=w867:T18[])  [unwired: 13 in, 1 out]
        n396 = Array Size(array=w867) -> (size(s)=w865:i32)
        n397 = call "Arange_Displays_V2.vi"("Display References"=w864, "Action"=w869, "Number of Channels"=w865, "Aspect Ratio (h/w)"=w870) -> ()  [unwired: 11 in, 1 out]
      }
      frame "Start Waveforms" {
        n398 = Unbundle By Name(w873) -> ("Scan Type"=w875:enum16{"Sample Scanning", "Beam Scanning"})
        n399 = case shown="\"Beam Scanning\"" w875 {
          tunnel: [w884 w885] -> w874
          frame "Sample Scanning", Default {
            n400 = local read "Unused Axis Voltage"() -> (w884:i16)
          }
          frame "Beam Scanning" {
            n401 = local read "Unused Axis Voltage"() -> (w885:i16)
          }
        }
        n402 = call "Initialize Waveforms V4.vi"("Image Acquisition Parameters"=w873) -> ("Waveform Data to FPGA"=w882:T19)  [unwired: 14 in]
        n403 = call "FPGA-7842R-Control V1.vi"("Waveform Data"=w882, "Action"=FPGA-7842R-Reference."Start Waveforms", "Image Acquisition Parameters"=w873, "Initialize"=w881) -> ("Initalized"=w877:bool)  [unwired: 11 in]
        n404 = call "FPGA-7842R-Control V1.vi"("Action"=FPGA-7842R-Reference."Unused Axis I16", "Initialize"=w877, "Unused Axis Offset (I16)"=w874) -> ("Initalized"=w876:bool)  [unwired: 12 in]
      }
      frame "Display" {
        w911 = u16 1 items=["Write", "Read"] ("Mode")
        n405 = call "Image_Actions_V1.vi"("Mode"=w911) -> ("Image REFs OUT"=w913:T18[])  [unwired: 13 in, 1 out]
        n406 = Array Size(array=w913) -> (size(s)=w909:i32)
        n407 = Decrement(x=w909) -> (x-1=w908:i32)
        n408 = for {
          N: 6 -> [_]
          tunnel: w908 -> [w947]
          tunnel: [w945] -> w912 mode=indexing
          i -> [w946]
          n409 = Greater Or Equal?(x=w947, y=w946) -> (x >= y?=w945:bool)
        }
        n410 = Obtain Notifier(name (unnamed)="Running", notification data type=FALSE) -> (notifier out=w916:refnum<notifier>)  [unwired: 2 in, 2 out]
        n411 = Index Array(array=w912, index #1=1 ("index"), index #2=2 ("index"), index #3=3 ("index"), index #4=4 ("index"), index #5=5 ("index")) -> (element #1=w897:bool, element #2=w896:bool, element #3=w895:bool, element #4=w894:bool, element #5=w893:bool)
        n412 = Index Array(array=w913, index #1=0 ("index"), index #2=1 ("index"), index #3=2 ("index"), index #4=3 ("index"), index #5=4 ("index"), index #6=5 ("index")) -> (element #1=w892:T18, element #2=w891:T18, element #3=w890:T18, element #4=w889:T18, element #5=w888:T18, element #6=w887:T18)
        n413 = while {
          tunnel: w897 -> [w934]
          tunnel: w896 -> [w933]
          tunnel: w895 -> [w929]
          tunnel: w894 -> [w926]
          tunnel: w893 -> [w925]
          tunnel: w892 -> [w932]
          tunnel: w891 -> [w931]
          tunnel: w890 -> [w930]
          tunnel: w889 -> [w928]
          tunnel: w888 -> [w922]
          tunnel: w887 -> [w927]
          tunnel: w916 -> [w924]
          stop <- w923 stop-if-true
          n414 = Get Notifier Status(notifier=w924) -> (current notification=w923:bool)  [unwired: 1 in, 4 out]
          n415 = case shown="False" w934 {
            tunnel: w931 -> [_ w944]
            frame False {
            }
            frame True {
              n416 = call "IMAQ ImageToArray"("Image"=w944) -> ("Image Pixels (Float)"=→"Channel 2":sgl[][])  [unwired: 3 in, 4 out]
            }
          }
          n417 = case shown="False" w933 {
            tunnel: w930 -> [_ w942]
            frame False {
            }
            frame True {
              n418 = call "IMAQ ImageToArray"("Image"=w942) -> ("Image Pixels (Float)"=→"Channel 3":sgl[][])  [unwired: 3 in, 4 out]
            }
          }
          n419 = call "IMAQ ImageToArray"("Image"=w932) -> ("Image Pixels (Float)"=→"Channel 1":sgl[][])  [unwired: 3 in, 4 out]
          n420 = Wait (ms)(milliseconds to wait=u32 30) -> ()  [unwired: 1 out]
          n421 = case shown="False" w929 {
            tunnel: w928 -> [_ w940]
            frame False {
            }
            frame True {
              n422 = call "IMAQ ImageToArray"("Image"=w940) -> ("Image Pixels (Float)"=→"Channel 4":sgl[][])  [unwired: 3 in, 4 out]
            }
          }
          n423 = case shown="False" w926 {
            tunnel: w922 -> [_ w938]
            frame False {
            }
            frame True {
              n424 = call "IMAQ ImageToArray"("Image"=w938) -> ("Image Pixels (Float)"=→"Channel 5":sgl[][])  [unwired: 3 in, 4 out]
            }
          }
          n425 = case shown="False" w925 {
            tunnel: w927 -> [_ w936]
            frame False {
            }
            frame True {
              n426 = call "IMAQ ImageToArray"("Image"=w936) -> ("Image Pixels (Float)"=→"Channel 6":sgl[][])  [unwired: 3 in, 4 out]
            }
          }
        }
      }
      frame "Stop Waveforms" {
        n427 = call "FPGA-7842R-Control V1.vi"("Action"=FPGA-7842R-Reference."Stop Waveforms", "Initialize"=w950) -> ("Initalized"=w949:bool)  [unwired: 13 in]
      }
      frame "Stop Acquisition" {
        n428 = call "FPGA-7842R-Control V1.vi"("Action"=FPGA-7842R-Reference."Laser Control", "Laser Controls"=T4 {"STED Power (V)"=0.0, "590 Power (V)"=0.0, "STED"=FALSE, "640 nm"=FALSE, "590 nm"=FALSE, "485 nm"=FALSE, "Manual Control"=FALSE} ("Laser Controls 2"), "Initialize"=TRUE) -> ()  [unwired: 12 in, 1 out]
      }
      frame "Start FPGA Acquisition" {
        n429 = Unbundle By Name(w961) -> ("Scan Type"=w960:enum16{"Sample Scanning", "Beam Scanning"})
        n430 = case shown="\"Sample Scanning\", Default" w960 {
          tunnel: w961 -> [w966 w974]
          tunnel: w959 -> [w965 w972]
          frame "Sample Scanning", Default {
            n431 = vi-ref "FPGA Sample Scanning V1.vi"() -> (w969:refnum<vi>)
            n432 = property class="VI Interface Type 0"(reference=w969) -> ("Path"=w967:path)  [unwired: 1 in, 2 out]
            n433 = Open VI Reference(type specifier VI Refnum (for type only)=w969, vi path=w967, options=128) -> (vi reference=w970:refnum<vi>)  [unwired: 3 in, 1 out]
            n434 = call-by-ref "Start Asynchronous Call"(reference=w970, "Detectors"=w965, "Image Acquisition Parameters"=w966) -> (reference out=w971:refnum<vi>)  [unwired: 2 in, 1 out]
            n435 = Close Reference(reference=w971) -> ()  [unwired: 1 in, 1 out]
          }
          frame "Beam Scanning" {
            n436 = vi-ref "FPGA Beam Scanning V1.vi"() -> (w977:refnum<vi>)
            n437 = property class="VI Interface Type 0"(reference=w977) -> ("Path"=w975:path)  [unwired: 1 in, 2 out]
            n438 = Open VI Reference(type specifier VI Refnum (for type only)=w977, vi path=w975, options=128) -> (vi reference=w973:refnum<vi>)  [unwired: 3 in, 1 out]
            n439 = call-by-ref "Start Asynchronous Call"(reference=w973, "Detectors"=w972, "Image Acquisition Parameters"=w974) -> (reference out=w978:refnum<vi>)  [unwired: 2 in, 1 out]
            n440 = Close Reference(reference=w978) -> ()  [unwired: 1 in, 1 out]
          }
        }
      }
    }
  }
